vi "数据编码.vi"(0 "table输入":string(combo), 1 "仪器参数上传时间":enum16{"精确到小时", "原始时间"}(ring), 5 "错误常量 2":errorcluster caption="错误输入", 7 "仪器参数":string[](array[string]), 9 "QN":string, 11 "参数":string, 13 "MN":string, 14 "PW":string) -> (4 "错误常量":errorcluster caption="错误输出", 15 "通讯包字符串":string)   [LabVIEW 2016, in "数据传输系统-06.lvlib"]
panel:
  out "核查数据发送次数":i32
  out "小时数据发送次数":i32
  out "长度":i32
  in  "数据块":T1
  out "通讯包":T2={"包头（2）"="##", "数据段长度（4）"="", "数据段"="", "CRC校验"="", "包尾"=""}
  # "范例代码：\n\n##0101QN=20160801085857223;ST=32;CN=1062;PW=100000;MN=010000A8900016F000169DC0;Flag=5\n;CP=&&RtdInterval=30&&1C80\\r\\n"
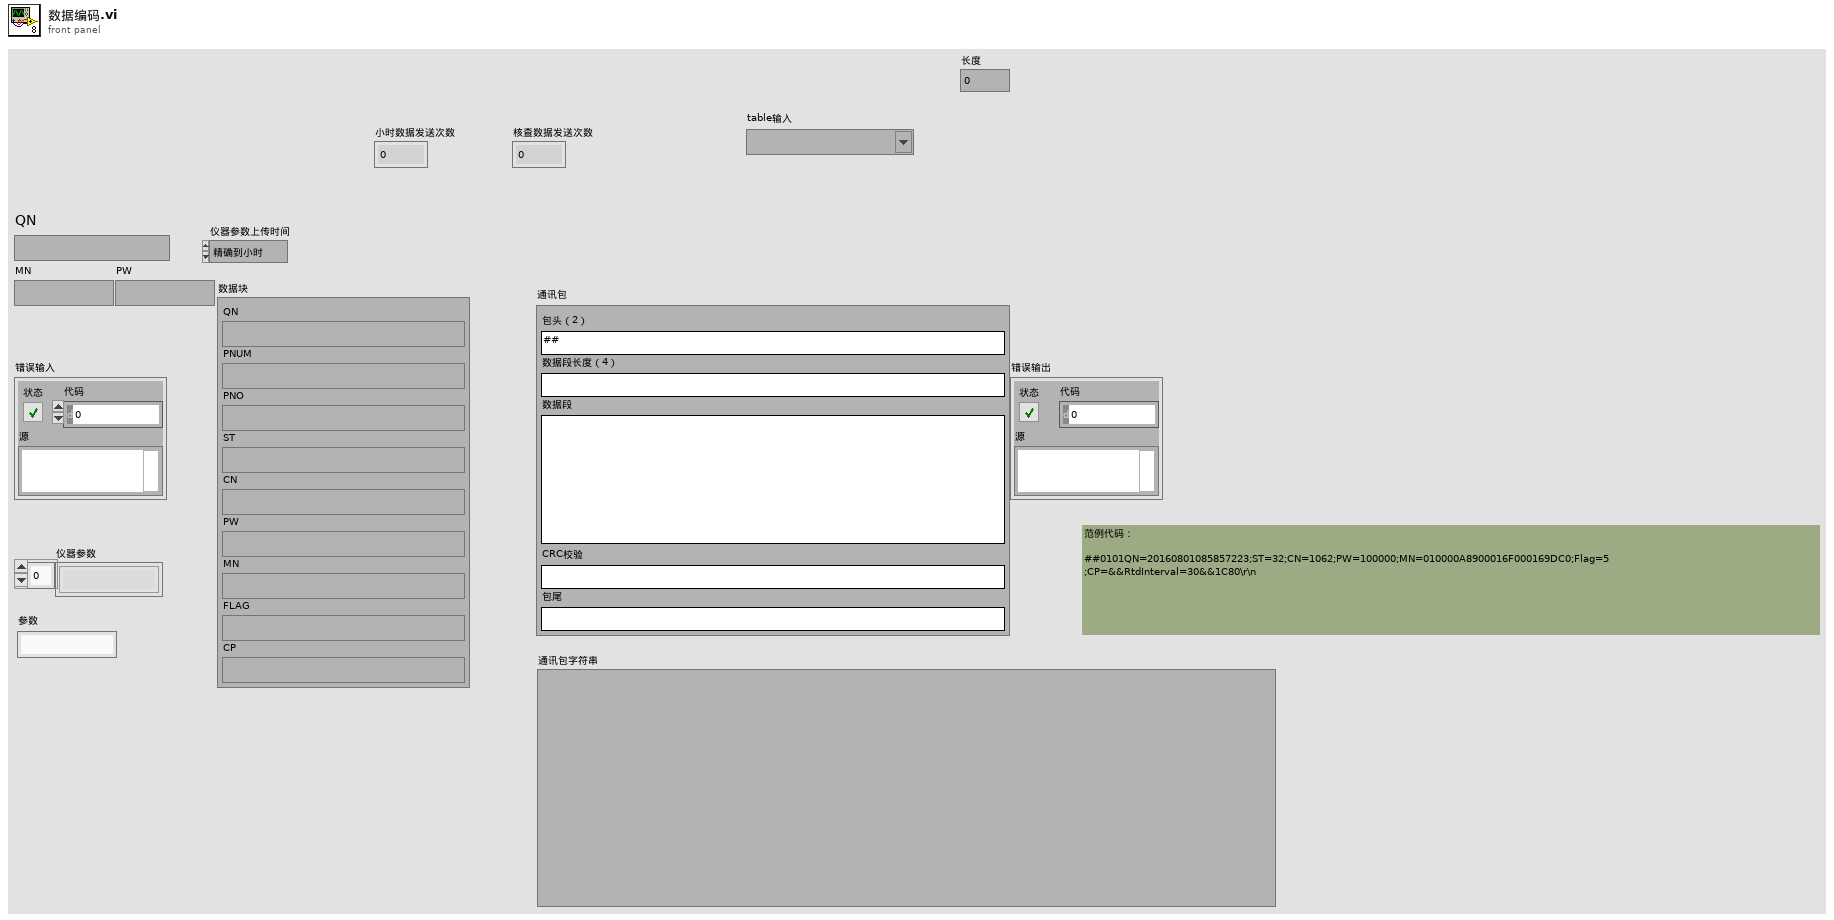
[diagram p1: front panel]
types:
  T1 = cluster{"QN":string, "ST":string, "CN":string, "PW":string, "MN":string, "FLAG":string, "PNUM":string, "PNO":string, "CP":string}
  T2 = cluster{"包头（2）":string, "数据段长度（4）":string, "数据段":string, "CRC校验":string, "包尾":string}
  T3 = cluster{"PH":string[][], "CODCr":string[][], "氨氮":string[][], "CODMn":string[][], "总氮":string[][], "总磷":string[][], "电导率":string[][], "水温":string[][], "DO":string[][], "浊度":string[][], "叶绿素":string[][], "藻密度":string[][], "铜":string[][], "盐度":string[][], "水位":string[][], "流速":string[][], "瞬时流量":string[][], "累积流量":string[][], "亚硝酸盐":string[][], "硫化物":string[][], "ORP":string[][], "铅":string[][], "镉":string[][], "锌":string[][], "镍":string[][], "锰":string[][], "汞":string[][], "气温":string[][], "气压":string[][], "风速":string[][], "风向":string[][], "盐度 2":string[][], "磷酸盐":string[][], "硝氮":string[][], "氟化物":string[][], "挥发酚":string[][], "氯化物":string[][]}
  T4 = enum16{"小时数据", "实时数据", "平行样测试", "集成干预测试", "加标回收测试", "核查数据", "空白零点跨度数据", "提取小时数据", "提取实时数据"}
  T5 = enum16{"小时数据", "实时数据", "平行样测试", "集成干预测试", "加标回收测试", "核查数据", "空白零点跨度数据", "提取小时数据", "提取实时数据", "操作日志"}
  T6 = enum16{"小时数据", "实时数据", "平行样测试", "集成干预测试", "加标回收测试", "核查数据", "空白零点跨度数据", "提取小时数据", "提取实时数据", "操作日志", "仪器参数", "3090仪器参数", "提取仪器参数", "报警信息"}
  T7 = cluster{"CODMn固件信息":string, "氨氮固件信息":string, "总磷固件信息":string, "总氮固件信息":string, "CODCr固件信息":string}
  T8 = typedef "数据传输系统-06.lvlib/应用环境.ctl" = enum16{"STD", "GB212", "婉仪平台"}
  T9 = cluster{"CODMn":dbl, "CODCr":dbl, "DO":dbl, "铜":dbl, "PH":dbl, "氨氮":dbl, "比电导率":dbl, "水温":dbl, "COD":dbl, "浊度":dbl, "总氮":dbl, "总磷":dbl, "叶绿素a":dbl, "藻密度":dbl, "水位":dbl, "流速":dbl, "瞬时流量":dbl, "累积流量":dbl, "亚硝酸盐":dbl, "硫化物":dbl, "ORP":dbl, "铅":dbl, "镉":dbl, "锌":dbl, "镍":dbl, "锰":dbl, "汞":dbl, "气温":dbl, "气压":dbl, "风速":dbl, "风向":dbl, "盐度":dbl, "磷酸盐":dbl, "硝氮":dbl, "氟化物":dbl, "挥发酚":dbl, "氯化物":dbl}
  T10 = cluster{"CODMn":string, "CODCr":string, "DO":string, "铜":string, "PH":string, "氨氮":string, "比电导率":string, "水温":string, "COD":string, "浊度":string, "总氮":string, "总磷":string, "叶绿素a":string, "藻密度":string, "水位":string, "流速":string, "瞬时流量":string, "累积流量":string, "亚硝酸盐":string, "硫化物":string, "ORP":string, "铅":string, "镉":string, "锌":string, "镍":string, "锰":string, "汞":string, "气温":string, "气压":string, "风速":string, "风向":string, "盐度":string, "磷酸盐":string, "硝氮":string, "氟化物":string, "挥发酚":string, "氯化物":string}
  T11 = typedef "LVDateTimeRec.ctl" = cluster{"秒数的小数部分":dbl, "秒":i32, "分":i32, "时":i32, "日":i32, "月":i32, "年":i32, "天数（周）":i32, "天数（年）":i32, "DST":i32}
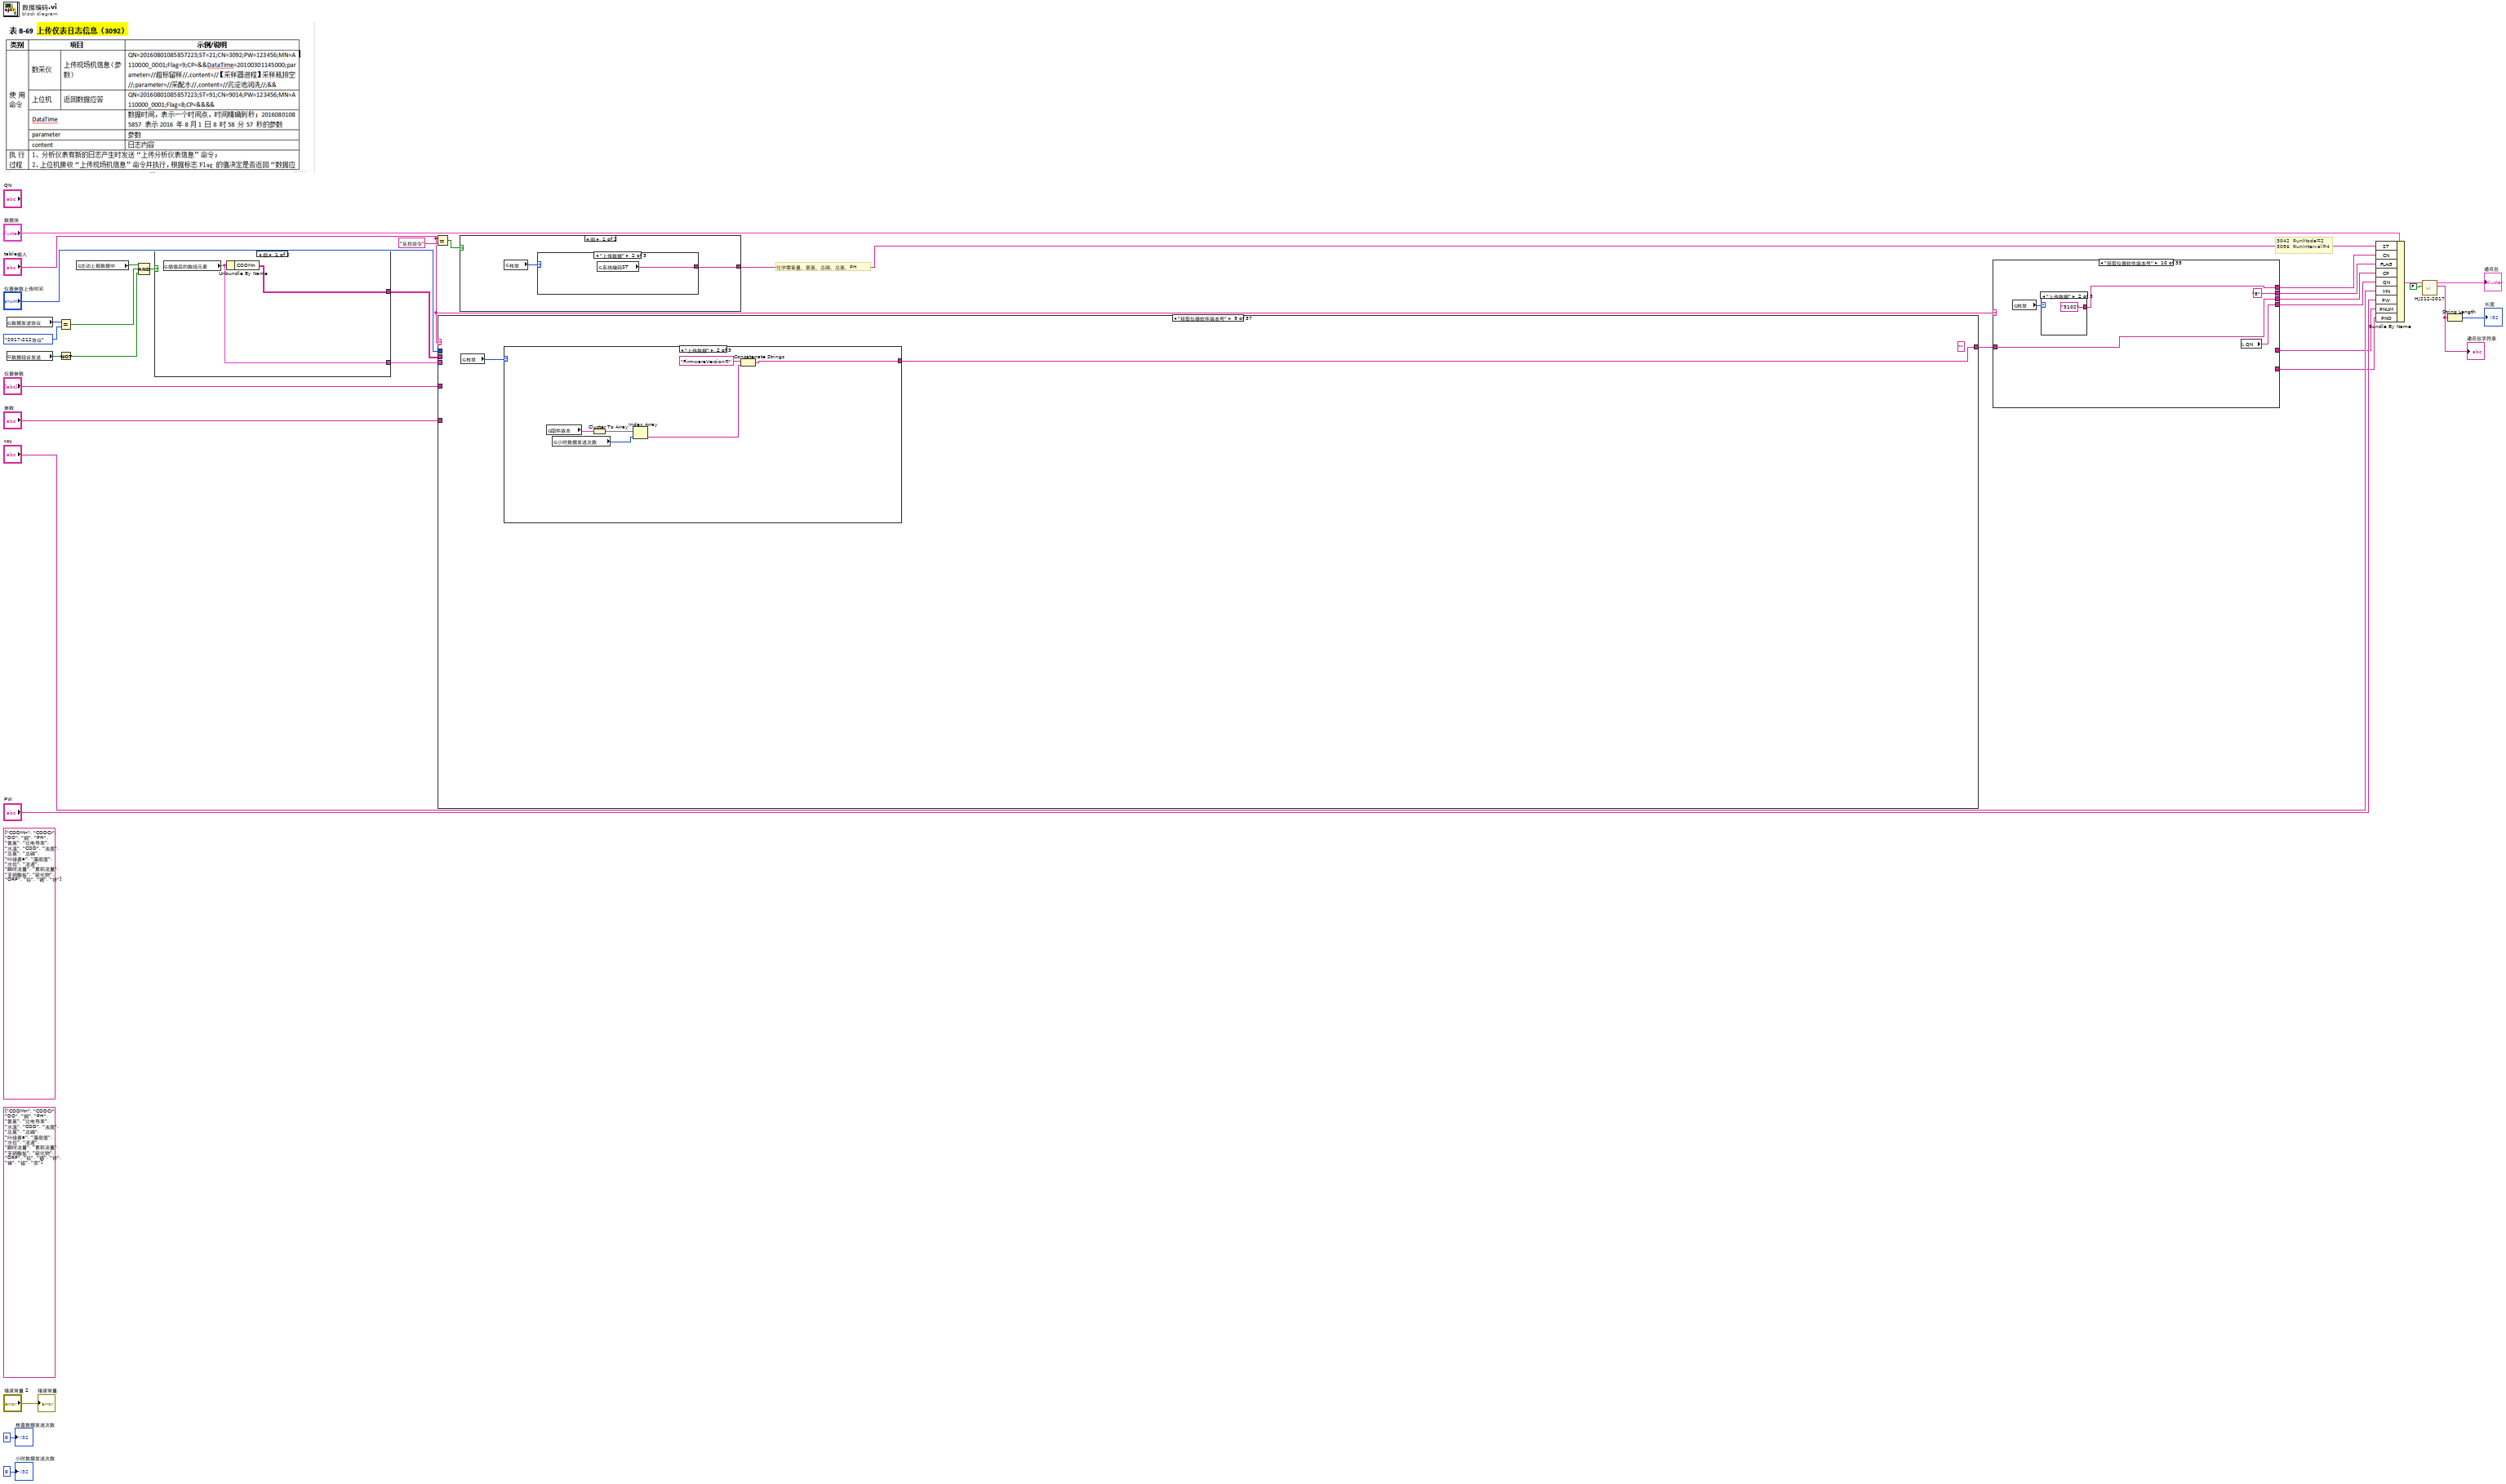
[diagram p0: block diagram]
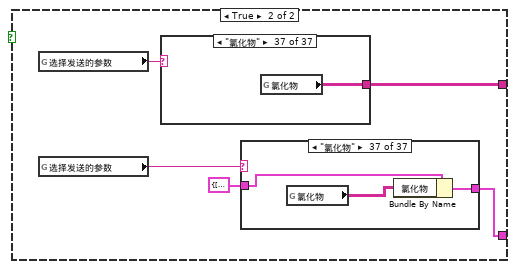
[diagram p2: hidden frame]
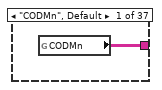
[diagram p3: hidden frame]
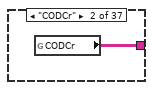
[diagram p4: hidden frame]
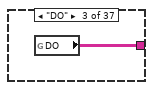
[diagram p5: hidden frame]
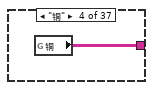
[diagram p6: hidden frame]
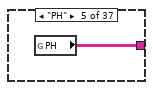
[diagram p7: hidden frame]
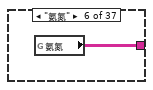
[diagram p8: hidden frame]
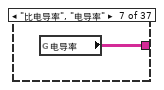
[diagram p9: hidden frame]
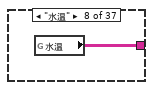
[diagram p10: hidden frame]
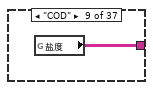
[diagram p11: hidden frame]
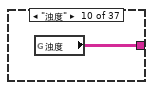
[diagram p12: hidden frame]
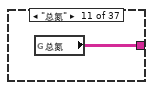
[diagram p13: hidden frame]
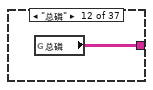
[diagram p14: hidden frame]
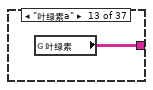
[diagram p15: hidden frame]
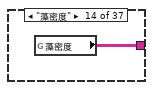
[diagram p16: hidden frame]
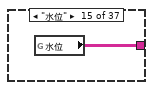
[diagram p17: hidden frame]
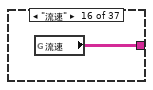
[diagram p18: hidden frame]
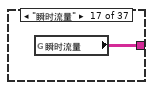
[diagram p19: hidden frame]
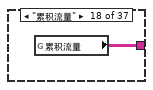
[diagram p20: hidden frame]
diagram:
  (unwired) string[] ["CODMn", "CODCr", "DO", "铜", "PH", "氨氮", "比电导率", "水温", "COD", "浊度", "总氮", "总磷", "叶绿素a", "藻密度", "水位", "流速", "瞬时流量", "累积流量", "亚硝酸盐", "硫化物", "ORP", "铅", "镉", "锌"] ("数组")
  (unwired) string[] ["CODMn", "CODCr", "DO", "铜", "PH", "氨氮", "比电导率", "水温", "COD", "浊度", "总氮", "总磷", "叶绿素a", "藻密度", "水位", "流速", "瞬时流量", "累积流量", "亚硝酸盐", "硫化物", "ORP", "铅", "镉", "锌", "镍", "锰", "汞"] ("数组")
  # "化学需氧量、氨氮、总磷、总氮、PH"
  # "3042  RunMode=2\n3056  RunInterval=4"
  n1 = global read "断电保存全局.vi" "数据发送协议"() -> (w11:enum16{"2005-212协议", "2017-212协议"})
  n2 = global read "断电保存全局.vi" "数据组合发送"() -> (w13:bool)
  n3 = Equal?(x=w11, y=enum16{"2005-212协议", "2017-212协议"}."2017-212协议" ("数据发送版本")) -> (x = y?=w14:bool)
  n4 = Not(x=w13) -> (.not. x?=w12:bool)
  n5 = global read "全局 数据发送重叠.vi" "主动上报数据中"() -> (w18:bool)
  n6 = Compound Arithmetic op=AND ("复合运算")(w18, w14, w12) -> (w15:bool)
  n7 = case shown="假" w15 {
    tunnel: [w36 w40] -> w9
    tunnel: [w35 w38] -> w7
    frame False {
      n8 = global read "插值后的新数组.vi" "插值后的数组元素"() -> (w36:T3)
      n9 = Unbundle By Name(w36) -> ("CODMn"=w35:string[][])
    }
    frame True {
      n10 = global read "全局 水样时间.vi" "选择发送的参数"() -> (w39:string)
      n11 = global read "全局 水样时间.vi" "选择发送的参数"() -> (w41:string)
      n12 = case shown="\"氯化物\"" w39 {
        tunnel: [w42 w43 w44 w45 w46 w47 w48 w49 w50 w51 w52 w53 w54 w55 w56 w57 w58 w59 w60 w61 w62 w63 w64 w65 w66 w67 w68 w69 w70 w71 w72 w73 w74 w75 w76 w77 w78] -> w38
        frame "CODMn", Default {
          n13 = global read "全局 所有参数.vi" "CODMn"() -> (w42:string[][])
        }
        frame "CODCr" {
          n14 = global read "全局 所有参数.vi" "CODCr"() -> (w43:string[][])
        }
        frame "DO" {
          n15 = global read "全局 所有参数.vi" "DO"() -> (w44:string[][])
        }
        frame "铜" {
          n16 = global read "全局 所有参数.vi" "铜"() -> (w45:string[][])
        }
        frame "PH" {
          n17 = global read "全局 所有参数.vi" "PH"() -> (w46:string[][])
        }
        frame "氨氮" {
          n18 = global read "全局 所有参数.vi" "氨氮"() -> (w47:string[][])
        }
        frame "比电导率", "电导率" {
          n19 = global read "全局 所有参数.vi" "电导率"() -> (w48:string[][])
        }
        frame "水温" {
          n20 = global read "全局 所有参数.vi" "水温"() -> (w49:string[][])
        }
        frame "COD" {
          n21 = global read "全局 所有参数.vi" "盐度"() -> (w50:string[][])
        }
        frame "浊度" {
          n22 = global read "全局 所有参数.vi" "浊度"() -> (w51:string[][])
        }
        frame "总氮" {
          n23 = global read "全局 所有参数.vi" "总氮"() -> (w52:string[][])
        }
        frame "总磷" {
          n24 = global read "全局 所有参数.vi" "总磷"() -> (w53:string[][])
        }
        frame "叶绿素a" {
          n25 = global read "全局 所有参数.vi" "叶绿素"() -> (w54:string[][])
        }
        frame "藻密度" {
          n26 = global read "全局 所有参数.vi" "藻密度"() -> (w55:string[][])
        }
        frame "水位" {
          n27 = global read "全局 所有参数.vi" "水位"() -> (w56:string[][])
        }
        frame "流速" {
          n28 = global read "全局 所有参数.vi" "流速"() -> (w57:string[][])
        }
        frame "瞬时流量" {
          n29 = global read "全局 所有参数.vi" "瞬时流量"() -> (w58:string[][])
        }
        frame "累积流量" {
          n30 = global read "全局 所有参数.vi" "累积流量"() -> (w59:string[][])
        }
        frame "亚硝氮" {
          n31 = global read "全局 所有参数.vi" "亚硝酸盐"() -> (w60:string[][])
        }
        frame "硫化物" {
          n32 = global read "全局 所有参数.vi" "硫化物"() -> (w61:string[][])
        }
        frame "ORP" {
          n33 = global read "全局 所有参数.vi" "ORP"() -> (w62:string[][])
        }
        frame "铅" {
          n34 = global read "全局 所有参数.vi" "铅"() -> (w63:string[][])
        }
        frame "镉" {
          n35 = global read "全局 所有参数.vi" "镉"() -> (w64:string[][])
        }
        frame "锌" {
          n36 = global read "全局 所有参数.vi" "锌"() -> (w65:string[][])
        }
        frame "镍" {
          n37 = global read "全局 所有参数.vi" "镍"() -> (w66:string[][])
        }
        frame "锰" {
          n38 = global read "全局 所有参数.vi" "锰"() -> (w67:string[][])
        }
        frame "汞" {
          n39 = global read "全局 所有参数.vi" "汞"() -> (w68:string[][])
        }
        frame "气温" {
          n40 = global read "全局 所有参数.vi" "气温"() -> (w69:string[][])
        }
        frame "气压" {
          n41 = global read "全局 所有参数.vi" "气压"() -> (w70:string[][])
        }
        frame "风速" {
          n42 = global read "全局 所有参数.vi" "风速"() -> (w71:string[][])
        }
        frame "风向" {
          n43 = global read "全局 所有参数.vi" "风向"() -> (w72:string[][])
        }
        frame "盐度" {
          n44 = global read "全局 所有参数.vi" "盐度 2"() -> (w73:string[][])
        }
        frame "磷酸盐" {
          n45 = global read "全局 所有参数.vi" "磷酸盐"() -> (w74:string[][])
        }
        frame "硝氮" {
          n46 = global read "全局 所有参数.vi" "硝氮"() -> (w75:string[][])
        }
        frame "氟化物" {
          n47 = global read "全局 所有参数.vi" "氟化物"() -> (w76:string[][])
        }
        frame "挥发酚" {
          n48 = global read "全局 所有参数.vi" "挥发酚"() -> (w77:string[][])
        }
        frame "氯化物" {
          n49 = global read "全局 所有参数.vi" "氯化物"() -> (w78:string[][])
        }
      }
      n50 = case shown="\"氯化物\"" w41 {
        tunnel: T3 {"PH"=[], "CODCr"=[], "氨氮"=[], "CODMn"=[], "总氮"=[], "总磷"=[], "电导率"=[], "水温"=[], "DO"=[], "浊度"=[], "叶绿素"=[], "藻密度"=[], "铜"=[], "盐度"=[], "水位"=[], "流速"=[], "瞬时流量"=[], "累积流量"=[], "亚硝酸盐"=[], "硫化物"=[], "ORP"=[], "铅"=[], "镉"=[], "锌"=[], "镍"=[], "锰"=[], "汞"=[], "气温"=[], "气压"=[], "风速"=[], "风向"=[], "盐度 2"=[], "磷酸盐"=[], "硝氮"=[], "氟化物"=[], "挥发酚"=[], "氯化物"=[]} ("插值后的数组元素") -> [w80 w84 w87 w90 w93 w96 w99 w102 w105 w108 w111 w114 w117 w119 w123 w126 w128 w131 w134 w137 w140 w143 w146 w149 w152 w155 w158 w161 w164 w167 w170 w173 w176 w179 w182 w185 w188]
        tunnel: [w79 w82 w85 w88 w91 w94 w98 w101 w103 w106 w109 w112 w115 w118 w121 w124 w127 w130 w133 w136 w139 w142 w145 w148 w151 w154 w157 w160 w163 w166 w169 w172 w175 w178 w181 w184 w187] -> w40
        frame "CODMn", Default {
          n51 = global read "全局 所有参数.vi" "CODMn"() -> (w81:string[][])
          n52 = Bundle By Name(cluster=w80, "CODMn"=w81) -> (w79:T3)
        }
        frame "CODCr" {
          n53 = global read "全局 所有参数.vi" "CODCr"() -> (w83:string[][])
          n54 = Bundle By Name(cluster=w84, "CODCr"=w83) -> (w82:T3)
        }
        frame "DO" {
          n55 = global read "全局 所有参数.vi" "DO"() -> (w86:string[][])
          n56 = Bundle By Name(cluster=w87, "DO"=w86) -> (w85:T3)
        }
        frame "铜" {
          n57 = global read "全局 所有参数.vi" "铜"() -> (w89:string[][])
          n58 = Bundle By Name(cluster=w90, "铜"=w89) -> (w88:T3)
        }
        frame "PH" {
          n59 = global read "全局 所有参数.vi" "PH"() -> (w92:string[][])
          n60 = Bundle By Name(cluster=w93, "PH"=w92) -> (w91:T3)
        }
        frame "氨氮" {
          n61 = global read "全局 所有参数.vi" "氨氮"() -> (w95:string[][])
          n62 = Bundle By Name(cluster=w96, "氨氮"=w95) -> (w94:T3)
        }
        frame "比电导率", "电导率" {
          n63 = global read "全局 所有参数.vi" "电导率"() -> (w97:string[][])
          n64 = Bundle By Name(cluster=w99, "电导率"=w97) -> (w98:T3)
        }
        frame "水温" {
          n65 = global read "全局 所有参数.vi" "水温"() -> (w100:string[][])
          n66 = Bundle By Name(cluster=w102, "水温"=w100) -> (w101:T3)
        }
        frame "COD" {
          n67 = global read "全局 所有参数.vi" "盐度"() -> (w104:string[][])
          n68 = Bundle By Name(cluster=w105, "盐度"=w104) -> (w103:T3)
        }
        frame "浊度" {
          n69 = global read "全局 所有参数.vi" "浊度"() -> (w107:string[][])
          n70 = Bundle By Name(cluster=w108, "浊度"=w107) -> (w106:T3)
        }
        frame "总氮" {
          n71 = global read "全局 所有参数.vi" "总氮"() -> (w110:string[][])
          n72 = Bundle By Name(cluster=w111, "总氮"=w110) -> (w109:T3)
        }
        frame "总磷" {
          n73 = global read "全局 所有参数.vi" "总磷"() -> (w113:string[][])
          n74 = Bundle By Name(cluster=w114, "总磷"=w113) -> (w112:T3)
        }
        frame "叶绿素a" {
          n75 = global read "全局 所有参数.vi" "叶绿素"() -> (w116:string[][])
          n76 = Bundle By Name(cluster=w117, "叶绿素"=w116) -> (w115:T3)
        }
        frame "藻密度" {
          n77 = global read "全局 所有参数.vi" "藻密度"() -> (w120:string[][])
          n78 = Bundle By Name(cluster=w119, "藻密度"=w120) -> (w118:T3)
        }
        frame "水位" {
          n79 = global read "全局 所有参数.vi" "水位"() -> (w122:string[][])
          n80 = Bundle By Name(cluster=w123, "水位"=w122) -> (w121:T3)
        }
        frame "流速" {
          n81 = global read "全局 所有参数.vi" "流速"() -> (w125:string[][])
          n82 = Bundle By Name(cluster=w126, "流速"=w125) -> (w124:T3)
        }
        frame "瞬时流量" {
          n83 = global read "全局 所有参数.vi" "瞬时流量"() -> (w129:string[][])
          n84 = Bundle By Name(cluster=w128, "瞬时流量"=w129) -> (w127:T3)
        }
        frame "累积流量" {
          n85 = global read "全局 所有参数.vi" "累积流量"() -> (w132:string[][])
          n86 = Bundle By Name(cluster=w131, "累积流量"=w132) -> (w130:T3)
        }
        frame "亚硝氮" {
          n87 = global read "全局 所有参数.vi" "亚硝酸盐"() -> (w135:string[][])
          n88 = Bundle By Name(cluster=w134, "亚硝酸盐"=w135) -> (w133:T3)
        }
        frame "硫化物" {
          n89 = global read "全局 所有参数.vi" "硫化物"() -> (w138:string[][])
          n90 = Bundle By Name(cluster=w137, "硫化物"=w138) -> (w136:T3)
        }
        frame "ORP" {
          n91 = global read "全局 所有参数.vi" "ORP"() -> (w141:string[][])
          n92 = Bundle By Name(cluster=w140, "ORP"=w141) -> (w139:T3)
        }
        frame "铅" {
          n93 = global read "全局 所有参数.vi" "铅"() -> (w144:string[][])
          n94 = Bundle By Name(cluster=w143, "铅"=w144) -> (w142:T3)
        }
        frame "镉" {
          n95 = global read "全局 所有参数.vi" "镉"() -> (w147:string[][])
          n96 = Bundle By Name(cluster=w146, "镉"=w147) -> (w145:T3)
        }
        frame "锌" {
          n97 = global read "全局 所有参数.vi" "锌"() -> (w150:string[][])
          n98 = Bundle By Name(cluster=w149, "锌"=w150) -> (w148:T3)
        }
        frame "镍" {
          n99 = global read "全局 所有参数.vi" "镍"() -> (w153:string[][])
          n100 = Bundle By Name(cluster=w152, "镍"=w153) -> (w151:T3)
        }
        frame "锰" {
          n101 = global read "全局 所有参数.vi" "锰"() -> (w156:string[][])
          n102 = Bundle By Name(cluster=w155, "锰"=w156) -> (w154:T3)
        }
        frame "汞" {
          n103 = global read "全局 所有参数.vi" "汞"() -> (w159:string[][])
          n104 = Bundle By Name(cluster=w158, "汞"=w159) -> (w157:T3)
        }
        frame "气温" {
          n105 = global read "全局 所有参数.vi" "气温"() -> (w162:string[][])
          n106 = Bundle By Name(cluster=w161, "气温"=w162) -> (w160:T3)
        }
        frame "气压" {
          n107 = global read "全局 所有参数.vi" "气压"() -> (w165:string[][])
          n108 = Bundle By Name(cluster=w164, "气压"=w165) -> (w163:T3)
        }
        frame "风速" {
          n109 = global read "全局 所有参数.vi" "风速"() -> (w168:string[][])
          n110 = Bundle By Name(cluster=w167, "风速"=w168) -> (w166:T3)
        }
        frame "风向" {
          n111 = global read "全局 所有参数.vi" "风向"() -> (w171:string[][])
          n112 = Bundle By Name(cluster=w170, "风向"=w171) -> (w169:T3)
        }
        frame "盐度" {
          n113 = global read "全局 所有参数.vi" "盐度 2"() -> (w174:string[][])
          n114 = Bundle By Name(cluster=w173, "盐度 2"=w174) -> (w172:T3)
        }
        frame "磷酸盐" {
          n115 = global read "全局 所有参数.vi" "磷酸盐"() -> (w177:string[][])
          n116 = Bundle By Name(cluster=w176, "磷酸盐"=w177) -> (w175:T3)
        }
        frame "硝氮" {
          n117 = global read "全局 所有参数.vi" "硝氮"() -> (w180:string[][])
          n118 = Bundle By Name(cluster=w179, "硝氮"=w180) -> (w178:T3)
        }
        frame "氟化物" {
          n119 = global read "全局 所有参数.vi" "氟化物"() -> (w183:string[][])
          n120 = Bundle By Name(cluster=w182, "氟化物"=w183) -> (w181:T3)
        }
        frame "挥发酚" {
          n121 = global read "全局 所有参数.vi" "挥发酚"() -> (w186:string[][])
          n122 = Bundle By Name(cluster=w185, "挥发酚"=w186) -> (w184:T3)
        }
        frame "氯化物" {
          n123 = global read "全局 所有参数.vi" "氯化物"() -> (w189:string[][])
          n124 = Bundle By Name(cluster=w188, "氯化物"=w189) -> (w187:T3)
        }
      }
    }
  }
  n125 = Equal?(x="table输入", y="反控命令") -> (x = y?=w24:bool)
  n126 = case shown="\"获取仪器软件版本号\"" "table输入" {
    tunnel: [w191 w198 w212 w254 w292 _ w306 w315 w322 w332 w343 w493 w524 w575 w623 w675 w704 w736 w767 w793 w822 w851 w888 w921 w954 w993 w1154 w1196 w1357 w1385 w1408 w1441 w1464 w1475 w1483 w1493 w1503] -> w19
    tunnel: w7 -> [_ _ _ _ _ _ _ _ _ _ w340 w492 _ _ _ w674 w705 w731 w762 w794 w821 w850 w887 _ _ _ _ _ w1356 _ w1407 _ _ _ _ _ _]
    tunnel: w9 -> [_ _ _ _ _ _ _ _ _ _ w341 w494 _ _ _ w670 w700 w732 w763 w792 w820 w849 w883 _ _ _ _ _ w1352 w1383 w1403 _ _ _ _ _ _]
    tunnel: "仪器参数" -> [_ _ _ _ _ _ _ _ _ _ _ _ _ _ _ _ _ _ _ _ _ _ _ _ _ w989 w1152 w1192 _ _ _ _ _ _ _ _ _]
    tunnel: "参数" -> [_ _ _ _ _ _ _ _ _ _ _ _ _ _ _ _ _ _ _ _ _ _ _ _ _ w991 _ w1194 _ _ _ _ _ _ _ _ _]
    tunnel: "仪器参数上传时间" -> [_ _ _ _ _ _ _ _ _ _ _ _ _ _ _ _ _ _ _ _ _ _ _ _ _ w988 w1151 w1191 _ _ _ _ _ _ _ _ _]
    frame "反控命令" {
      n127 = global read "全局 反控命令枚举.vi" "反控命令枚举"() -> (w190:enum16{"返回请求应答", "返回执行结果"})
      n128 = case shown="\"返回执行结果\"" w190 {
        tunnel: ["QnRtn=1" w194] -> w191
        frame "返回请求应答", Default {
        }
        frame "返回执行结果" {
          n129 = global read "全局 反控命令枚举.vi" "执行结果定义"() -> (w195:u16)
          n130 = Number To Decimal String(number=w195) -> (decimal integer string=w193:string)  [unwired: 1 in]
          n131 = Concatenate Strings("ExeRtn=", w193) -> (w194:string)
        }
      }
    }
    frame "超标留样返回" {
      n132 = global read "全局1.vi" "枚举"() -> (w197:enum16{"返回请求应答", "上传数据", "返回执行结果"})
      n133 = case shown="\"返回执行结果\"" w197 {
        tunnel: ["QnRtn=1" w200 "ExeRtn=1"] -> w198
        frame "返回请求应答", Default {
        }
        frame "上传数据" {
          n134 = global read "全局1.vi" "register values"() -> (w209:u16[])
          n135 = Get Date/Time In Seconds() -> (seconds since 1Jan1904=w207:timestamp)
          n136 = Index Array(array=w209, index=7 ("索引")) -> (element=w202:u16)
          n137 = Format Date/Time String(time format string (%c)="%Y%m%d%H%M%S" ("时间格式字符串(%c)"), seconds (now)=w207) -> (date/time string=w205:string)  [unwired: 1 in]
          n138 = Number To Decimal String(number=w202) -> (decimal integer string=w203:string)  [unwired: 1 in]
          n139 = Format Into String(format string="VaseNo=%s" ("格式字符串"), w203) -> (resulting string=w201:string)  [unwired: 2 in, 1 out]
          n140 = Format Into String(format string="DataTime=%s;%s" ("格式字符串"), w205, w201) -> (resulting string=w200:string)  [unwired: 2 in, 1 out]
        }
        frame "返回执行结果" {
        }
      }
    }
    frame "提取经纬度环境信息" {
      # "BDS纬度"
      # "BDS纬度"
      # "GPS纬度"
      # "GPS经度"
      # "湿度"
      # "温度"
      # "电压"
      # "时间"
      n141 = global read "全局1.vi" "枚举"() -> (w213:enum16{"返回请求应答", "上传数据", "返回执行结果"})
      n142 = case shown="\"上传数据\"" w213 {
        tunnel: ["QnRtn=1" w226 "ExeRtn=1"] -> w212
        frame "返回请求应答", Default {
        }
        frame "上传数据" {
          n143 = global read "全局 环境参数.vi" "环境参数"() -> (w216:string[][])
          n144 = global read "全局 环境参数.vi" "columns输出"() -> (w223:string[])
          n145 = Index Array(array=w216, index (row)=0 ("索引 (行)")) -> (element=w219:string[])  [unwired: 1 in]
          n146 = Get Date/Time In Seconds() -> (seconds since 1Jan1904=w228:timestamp)
          n147 = Array Subset(array=w223, index=1 ("索引")) -> (w224:string[])  [unwired: 1 in]
          n148 = for {
            tunnel: w224 -> [w232] mode=indexing
            tunnel: [w231] -> w225 mode=indexing
            n149 = case shown="\"BDS经度\"" w232 {
              tunnel: ["" "Volt=%s;" "Temp=%s;" ("格式字符串") "Hum=%s;" ("格式字符串") "Lng=%s;" "Lat=%s;" "Lng2=%s;" "Lat2=%s;"] -> w231
              frame "假", Default {
              }
              frame "电压" {
              }
              frame "室温" {
              }
              frame "湿度" {
              }
              frame "GPS经度" {
              }
              frame "GPS纬度" {
              }
              frame "BDS经度" {
              }
              frame "BDS纬度" {
              }
            }
          }
          n150 = Format Date/Time String(time format string (%c)="%Y%m%d%H%M%S" ("时间格式字符串(%c)"), seconds (now)=w228) -> (date/time string=w227:string)  [unwired: 1 in]
          n151 = Array Subset(array=w219, index=1 ("索引")) -> (w221:string[])  [unwired: 1 in]
          n152 = for {
            shift-right: [w246] -> w215
            shift-left: "" -> [w245]
            tunnel: w225 -> [w244] mode=indexing
            tunnel: w221 -> [w242] mode=indexing
            n153 = Empty String/Path?(string/path=w242) -> (empty?=w248:bool)
            n154 = Fract/Exp String To Number(string=w242) -> (number=w243:dbl)  [unwired: 3 in, 1 out]
            n155 = Number To Fractional String(number=w243) -> (F-format string=w241:string)  [unwired: 3 in]
            n156 = case shown="假" w248 {
              tunnel: [w251 w252] -> w247
              tunnel: w244 -> [w250 _]
              tunnel: w241 -> [w249 _]
              tunnel: w241 -> [_ w252]
              frame False {
                n157 = Format Into String(format string=w250, w249) -> (resulting string=w251:string)  [unwired: 2 in, 1 out]
              }
              frame True {
              }
            }
            n158 = Concatenate Strings(w245, w247) -> (w246:string)
          }
          n159 = Format Into String(format string="DataTime=%s;%s" ("格式字符串"), w227, w215) -> (resulting string=w226:string)  [unwired: 2 in, 1 out]
        }
        frame "返回执行结果" {
        }
      }
    }
    frame "提取现场系统信息" {
      n160 = global read "全局1.vi" "枚举"() -> (w255:enum16{"返回请求应答", "上传数据", "返回执行结果"})
      n161 = case shown="\"上传数据\"" w255 {
        tunnel: ["QnRtn=1" w289 "ExeRtn=1"] -> w254
        frame "返回请求应答", Default {
        }
        frame "上传数据" {
          n162 = global read "全局1.vi" "register values"() -> (w288:u16[])
          n163 = global read "全局1.vi" "系统信息"() -> (w270:u16[])
          n164 = Get Date/Time In Seconds() -> (seconds since 1Jan1904=w275:timestamp)
          n165 = Format Date/Time String(time format string (%c)="%Y%m%d%H%M%S%u" ("时间格式字符串(%c)"), seconds (now)=w275) -> (date/time string=w278:string)  [unwired: 1 in]
          n166 = Number To Decimal String(number=w270) -> (decimal integer string=w269:string[])  [unwired: 1 in]
          n167 = Index Array(array=w288, index #1=0 ("索引"), index #2=6 ("索引")) -> (element #1=w284:u16, element #2=w272:u16)
          n168 = Number To Decimal String(number=w284) -> (decimal integer string=w286:string)  [unwired: 1 in]
          n169 = Number To Decimal String(number=w272) -> (decimal integer string=w281:string)  [unwired: 1 in]
          n170 = Index Array(array=w269) -> (element #1=w267:string, element #2=w264:string, element #3=w261:string, element #4=w258:string)  [unwired: 4 in]
          n171 = Search and Replace String(input string=w278, search string="." ("搜索字符串")) -> (result string=w274:string)  [unwired: 6 in, 3 out]
          n172 = Format Into String(format string="SystemTask=%s;" ("格式字符串"), w267) -> (resulting string=w266:string)  [unwired: 2 in, 1 out]
          n173 = Format Into String(format string="PumpState=%s;" ("格式字符串"), w264) -> (resulting string=w263:string)  [unwired: 2 in, 1 out]
          n174 = Format Into String(format string="AlgClean=%s;" ("格式字符串"), w261) -> (resulting string=w260:string)  [unwired: 2 in, 1 out]
          n175 = Format Into String(format string="SystemAlarm=0%s;" ("格式字符串"), w258) -> (resulting string=w257:string)  [unwired: 2 in, 1 out]
          n176 = Format Into String(format string="RunMode=%s;" ("格式字符串"), w286) -> (resulting string=w271:string)  [unwired: 2 in, 1 out]
          n177 = Format Into String(format string="RunInterval=%s;" ("格式字符串"), w281) -> (resulting string=w282:string)  [unwired: 2 in, 1 out]
          n178 = Format Into String(format string="SystemTime=%s;" ("格式字符串"), w274) -> (resulting string=w279:string)  [unwired: 2 in, 1 out]
          n179 = Concatenate Strings(w271, w263, w266, w260, w257, w282, w279) -> (w289:string)
        }
        frame "返回执行结果" {
        }
      }
    }
    frame "提取监测仪表时间" {
      n180 = global read "全局1.vi" "枚举"() -> (w291:enum16{"返回请求应答", "上传数据", "返回执行结果"})
      n181 = case shown="\"上传数据\"" w291 {
        tunnel: ["QnRtn=1" w304 "ExeRtn=1"] -> w292
        frame "返回请求应答", Default {
        }
        frame "上传数据" {
          n182 = global read "全局 提取仪器参数.vi" "仪器编码"() -> (w294:string)
          n183 = Format Into String(format string="PolId=%s;" ("格式字符串"), w294) -> (resulting string=w302:string)  [unwired: 2 in, 1 out]
          n184 = Get Date/Time In Seconds() -> (seconds since 1Jan1904=w297:timestamp)
          n185 = Format Date/Time String(time format string (%c)="%Y%m%d%H%M%S%u" ("时间格式字符串(%c)"), seconds (now)=w297) -> (date/time string=w300:string)  [unwired: 1 in]
          n186 = Search and Replace String(input string=w300, search string="." ("搜索字符串")) -> (result string=w296:string)  [unwired: 6 in, 3 out]
          n187 = Format Into String(format string="SystemTime=%s;" ("格式字符串"), w296) -> (resulting string=w295:string)  [unwired: 2 in, 1 out]
          n188 = Concatenate Strings(w302, w295) -> (w304:string)
        }
        frame "返回执行结果" {
        }
      }
    }
    frame "心跳包", Default {
    }
    frame "提取数采仪时间" {
      (unwired) ""
      n189 = global read "全局1.vi" "枚举"() -> (w307:enum16{"返回请求应答", "上传数据", "返回执行结果"})
      n190 = case shown="\"上传数据\"" w307 {
        tunnel: ["QnRtn=1" w309 "ExeRtn=1"] -> w306
        frame "返回请求应答", Default {
        }
        frame "上传数据" {
          n191 = Get Date/Time In Seconds() -> (seconds since 1Jan1904=w313:timestamp)
          n192 = Format Date/Time String(time format string (%c)="%Y%m%d%H%M%S" ("时间格式字符串(%c)"), seconds (now)=w313) -> (date/time string=w310:string)  [unwired: 1 in]
          n193 = Concatenate Strings("SystemTime=", w310) -> (w309:string)
        }
        frame "返回执行结果" {
        }
      }
    }
    frame "获取软件版本号" {
      (unwired) ""
      n194 = global read "全局1.vi" "枚举"() -> (w316:enum16{"返回请求应答", "上传数据", "返回执行结果"})
      n195 = case shown="\"上传数据\"" w316 {
        tunnel: ["QnRtn=1" w319 "ExeRtn=1"] -> w315
        frame "返回请求应答", Default {
        }
        frame "上传数据" {
          n196 = global read "全局1.vi" "版本信息"() -> (w318:string)
          n197 = Concatenate Strings("Version=", w318) -> (w319:string)
        }
        frame "返回执行结果" {
        }
      }
    }
    frame "获取仪器软件版本号" {
      (unwired) ""
      n198 = global read "全局1.vi" "枚举"() -> (w323:enum16{"返回请求应答", "上传数据", "返回执行结果"})
      n199 = case shown="\"上传数据\"" w323 {
        tunnel: ["QnRtn=1" w329 "ExeRtn=1"] -> w322
        frame "返回请求应答", Default {
        }
        frame "上传数据" {
          n200 = global read "全局1.vi" "固件版本"() -> (w328:T7)
          n201 = global read "全局 小时数据发送次数.vi" "小时数据发送次数"() -> (w326:i32)
          n202 = Cluster To Array(cluster=w328) -> (array=w327:string[])
          n203 = Index Array(array=w327, index=w326) -> (element=w325:string)
          n204 = Concatenate Strings("FirmwareVersion=", w325) -> (w329:string)
        }
        frame "返回执行结果" {
        }
      }
    }
    frame "提取实时数据间隔" {
      (unwired) ""
      n205 = global read "全局1.vi" "枚举"() -> (w333:enum16{"返回请求应答", "上传数据", "返回执行结果"})
      n206 = case shown="\"上传数据\"" w333 {
        tunnel: ["QnRtn=1" w337 "ExeRtn=1"] -> w332
        frame "返回请求应答", Default {
        }
        frame "上传数据" {
          n207 = global read "实时数据发送间隔全局.vi" "实时数据发送间隔"() -> (w336:u32)
          n208 = Number To Decimal String(number=w336) -> (decimal integer string=w335:string)  [unwired: 1 in]
          n209 = Concatenate Strings("RtdInterval=", w335) -> (w337:string)
        }
        frame "返回执行结果" {
        }
      }
    }
    frame "实时数据" {
      # "包含质控数据主动上传"
      n210 = global read "全局 实时数据参数.vi" "实时数据参数"() -> (w342:string)
      n211 = case shown="\"集成干预测试\"" w342 {
        tunnel: [w346 w371 w396 w427 w451 w472] -> w343
        tunnel: w341 -> [w345 w370 w395 w425 w449 w470]
        tunnel: w340 -> [w344 w369 w394 w424 w448 w469]
        frame "水样测试", Default {
          n212 = global read "全局1.vi" "枚举"() -> (w347:enum16{"返回请求应答", "上传数据", "返回执行结果"})
          n213 = case shown="\"上传数据\"" w347 {
            tunnel: ["QnRtn=1" w365 "ExeRtn=1"] -> w346
            tunnel: w345 -> [_ w351 _]
            tunnel: w344 -> [_ w349 _]
            frame "返回请求应答", Default {
            }
            frame "上传数据" {
              n214 = call "数据发送组合-20200825 (子VI).vi"("枚举"=T4."实时数据", "插值后的数组元素"=w351) -> ("字符串"=w352:string)  [unwired: 9 in]
              n215 = global read "全局 小时数据发送次数.vi" "小时数据发送次数"() -> (w363:i32)
              n216 = Index Array(array=w349, index (row)=w363) -> (element=w362:string[])  [unwired: 1 in]
              n217 = Index Array(array=w362, index=0 ("索引")) -> (element=w360:string)
              n218 = call "规范时间戳.vi"("字符串"=w360) -> ("result string"=w358:string)  [unwired: 10 in]
              n219 = Empty String/Path?(string/path=w352) -> (empty?=w364:bool)
              n220 = Format Into String(format string="DataTime=%s;", w358) -> (resulting string=w357:string)  [unwired: 2 in, 1 out]
              n221 = Concatenate Strings(w357, w352) -> (w354:string)
              n222 = String Length(string=w354) -> (length=w356:i32)
              n223 = Decrement(x=w356) -> (x-1=w355:i32)
              n224 = String Subset(string=w354, length (rest)=w355) -> (substring=w353:string)  [unwired: 1 in]
              n225 = case shown="假" w364 {
                tunnel: [w366 ""] -> w365
                tunnel: w353 -> [w366 _]
                frame False {
                }
                frame True {
                }
              }
            }
            frame "返回执行结果" {
            }
          }
        }
        frame "平行样测试" {
          n226 = global read "全局1.vi" "枚举"() -> (w372:enum16{"返回请求应答", "上传数据", "返回执行结果"})
          n227 = case shown="\"上传数据\"" w372 {
            tunnel: ["QnRtn=1" w384 "ExeRtn=1"] -> w371
            tunnel: w369 -> [_ w378 _]
            tunnel: w370 -> [_ w375 _]
            frame "返回请求应答", Default {
            }
            frame "上传数据" {
              # "CODMn"
              n228 = call "数据发送组合-20200825 (子VI).vi"("枚举"=T4."平行样测试", "插值后的数组元素"=w375) -> ("字符串"=w374:string)  [unwired: 9 in]
              n229 = global read "全局 小时数据发送次数.vi" "小时数据发送次数"() -> (w377:i32)
              n230 = Index Array(array=w378, index (row)=w377) -> (element=w382:string[])  [unwired: 1 in]
              n231 = Index Array(array=w382, index=0 ("索引")) -> (element=w379:string)
              n232 = call "规范时间戳.vi"("字符串"=w379) -> ("result string"=w380:string)  [unwired: 10 in]
              n233 = Empty String/Path?(string/path=w379) -> (empty?=w383:bool)
              n234 = Format Into String(format string="DataTime=%s;%s" ("格式字符串"), w380, w374) -> (resulting string=w385:string)  [unwired: 2 in, 1 out]
              n235 = case shown="真" w383 {
                tunnel: [w389 ""] -> w384
                tunnel: w385 -> [w389 _]
                frame False {
                  n236 = global read "全局 小时数据发送次数.vi" "小时数据发送次数"() -> (w388:i32)
                  n237 = Increment(x=w388) -> (x+1=w387:i32)
                  n238 = global write "全局 小时数据发送次数.vi" "小时数据发送次数"(w387) -> ()
                }
                frame True {
                  n239 = global read "全局 小时数据发送次数.vi" "小时数据发送次数"() -> (w391:i32)
                  n240 = Increment(x=w391) -> (x+1=w390:i32)
                  n241 = global write "全局 小时数据发送次数.vi" "小时数据发送次数"(w390) -> ()
                }
              }
            }
            frame "返回执行结果" {
            }
          }
        }
        frame "集成干预测试" {
          n242 = global read "全局1.vi" "枚举"() -> (w397:enum16{"返回请求应答", "上传数据", "返回执行结果"})
          n243 = case shown="\"上传数据\"" w397 {
            tunnel: ["QnRtn=1" w410 "ExeRtn=1"] -> w396
            tunnel: w394 -> [_ w404 _]
            tunnel: w395 -> [_ w401 _]
            frame "返回请求应答", Default {
            }
            frame "上传数据" {
              # "CODMn"
              n244 = global read "全局 小时数据发送次数.vi" "小时数据发送次数"() -> (w403:i32)
              n245 = call "数据发送组合-20200825 (子VI).vi"("枚举"=T4."集成干预测试", "插值后的数组元素"=w401) -> ("字符串"=w400:string)  [unwired: 9 in]
              n246 = Index Array(array=w404, index (row)=w403) -> (element=w408:string[])  [unwired: 1 in]
              n247 = global read "断电保存全局.vi" "应用环境"() -> (w399:T8)
              n248 = Index Array(array=w408, index=0 ("索引")) -> (element=w405:string)
              n249 = case shown="\"GB212\", 默认" w399 {
                tunnel: [w414 w415] -> w406
                tunnel: w405 -> [w413 w416]
                frame "STD" {
                  n250 = call "规范时间戳.vi"("字符串"=w413) -> ("result string"=w414:string)  [unwired: 10 in]
                }
                frame "GB212", Default {
                  n251 = call "规范分钟数据时间戳.vi"("字符串"=w416) -> ("result string"=w415:string)  [unwired: 10 in]
                }
              }
              n252 = Empty String/Path?(string/path=w405) -> (empty?=w409:bool)
              n253 = Format Into String(format string="DataTime=%s;%s" ("格式字符串"), w406, w400) -> (resulting string=w411:string)  [unwired: 2 in, 1 out]
              n254 = case shown="假" w409 {
                tunnel: [w419 ""] -> w410
                tunnel: w411 -> [w419 _]
                frame False {
                  n255 = global read "全局 小时数据发送次数.vi" "小时数据发送次数"() -> (w418:i32)
                  n256 = Increment(x=w418) -> (x+1=w417:i32)
                  n257 = global write "全局 小时数据发送次数.vi" "小时数据发送次数"(w417) -> ()
                }
                frame True {
                  n258 = global read "全局 小时数据发送次数.vi" "小时数据发送次数"() -> (w421:i32)
                  n259 = Increment(x=w421) -> (x+1=w420:i32)
                  n260 = global write "全局 小时数据发送次数.vi" "小时数据发送次数"(w420) -> ()
                }
              }
            }
            frame "返回执行结果" {
            }
          }
        }
        frame "加标回收测试" {
          n261 = global read "全局1.vi" "枚举"() -> (w426:enum16{"返回请求应答", "上传数据", "返回执行结果"})
          n262 = case shown="\"上传数据\"" w426 {
            tunnel: ["QnRtn=1" w437 "ExeRtn=1"] -> w427
            tunnel: w424 -> [_ w432 _]
            tunnel: w425 -> [_ w434 _]
            frame "返回请求应答", Default {
            }
            frame "上传数据" {
              # "w01001-Check=63.0,w01001-WaterTime=20160801080000,w01001-Water=45.23,w01001-Chroma=1000,w01001-Volume=0.2,w01001-DVolume=200,w01003-Flag=N;"
              # "CODMn"
              n263 = global read "全局 小时数据发送次数.vi" "小时数据发送次数"() -> (w431:i32)
              n264 = call "加标回收数据组合 (子VI).vi"("小时数据发送次数"=w431, "数据"=w432, "污染物编码"="CODMn") -> ("datatime"=w430:string)  [unwired: 7 in, 1 out]
              n265 = call "规范时间戳.vi"("字符串"=w430) -> ("result string"=w439:string)  [unwired: 10 in]
              n266 = Empty String/Path?(string/path=w439) -> (empty?=w436:bool)
              n267 = call "数据发送组合-20200825 (子VI).vi"("枚举"=T4."加标回收测试", "插值后的数组元素"=w434) -> ("字符串"=w433:string)  [unwired: 9 in]
              n268 = Format Into String(format string="DataTime=%s;%s" ("格式字符串"), w439, w433) -> (resulting string=w438:string)  [unwired: 2 in, 1 out]
              n269 = case shown="真" w436 {
                tunnel: [w443 ""] -> w437
                tunnel: w438 -> [w443 _]
                frame False {
                  n270 = global read "全局 小时数据发送次数.vi" "小时数据发送次数"() -> (w442:i32)
                  n271 = Increment(x=w442) -> (x+1=w441:i32)
                  n272 = global write "全局 小时数据发送次数.vi" "小时数据发送次数"(w441) -> ()
                }
                frame True {
                  n273 = global read "全局 小时数据发送次数.vi" "小时数据发送次数"() -> (w445:i32)
                  n274 = Increment(x=w445) -> (x+1=w444:i32)
                  n275 = global write "全局 小时数据发送次数.vi" "小时数据发送次数"(w444) -> ()
                }
              }
            }
            frame "返回执行结果" {
            }
          }
        }
        frame "核查数据" {
          n276 = global read "全局1.vi" "枚举"() -> (w450:enum16{"返回请求应答", "上传数据", "返回执行结果"})
          n277 = case shown="\"上传数据\"" w450 {
            tunnel: ["QnRtn=1" w461 "ExeRtn=1"] -> w451
            tunnel: w449 -> [_ w454 _]
            tunnel: w448 -> [_ w453 _]
            frame "返回请求应答", Default {
            }
            frame "上传数据" {
              # "将非空数组的时间戳写入"
              n278 = global read "全局 小时数据发送次数.vi" "小时数据发送次数"() -> (w457:i32)
              n279 = Index Array(array=w453, index (row)=w457) -> (element=w460:string[])  [unwired: 1 in]
              n280 = call "数据发送组合-20200825 (子VI).vi"("枚举"=T4."核查数据", "插值后的数组元素"=w454) -> ("字符串"=w455:string)  [unwired: 9 in]
              n281 = Index Array(array=w460, index=0 ("索引")) -> (element=w459:string)
              n282 = call "规范分钟数据时间戳.vi"("字符串"=w459) -> ("result string"=w458:string)  [unwired: 10 in]
              n283 = Empty String/Path?(string/path=w458) -> (empty?=w463:bool)
              n284 = Format Into String(format string="DataTime=%s;%s" ("格式字符串"), w458, w455) -> (resulting string=w462:string)  [unwired: 2 in, 1 out]
              n285 = case shown="假" w463 {
                tunnel: [w466 ""] -> w461
                tunnel: w462 -> [w466 _]
                frame False {
                }
                frame True {
                }
              }
            }
            frame "返回执行结果" {
            }
          }
        }
        frame "空白测试", "跨度核查" {
          n286 = global read "全局1.vi" "枚举"() -> (w471:enum16{"返回请求应答", "上传数据", "返回执行结果"})
          n287 = case shown="\"上传数据\"" w471 {
            tunnel: ["QnRtn=1" w482 "ExeRtn=1"] -> w472
            tunnel: w470 -> [_ w476 _]
            tunnel: w469 -> [_ w474 _]
            frame "返回请求应答", Default {
            }
            frame "上传数据" {
              n288 = global read "全局 小时数据发送次数.vi" "小时数据发送次数"() -> (w480:i32)
              n289 = call "数据发送组合-20200825 (子VI).vi"("枚举"=T4."空白零点跨度数据", "插值后的数组元素"=w476) -> ("字符串"=w475:string)  [unwired: 9 in]
              n290 = Index Array(array=w474, index (row)=w480) -> (element=w486:string[])  [unwired: 1 in]
              n291 = Index Array(array=w486, index #1=0 ("索引"), index #2=3 ("索引"), index #3=7 ("索引")) -> (element #1=w479:string)  [unwired: 2 out]
              n292 = call "规范小时时间戳.vi"("字符串"=w479) -> ("result string"=w478:string)  [unwired: 10 in]
              n293 = Empty String/Path?(string/path=w478) -> (empty?=w483:bool)
              n294 = Format Into String(format string="DataTime=%s;%s" ("格式字符串"), w478, w475) -> (resulting string=w481:string)  [unwired: 2 in, 1 out]
              n295 = case shown="假" w483 {
                tunnel: [w489 ""] -> w482
                tunnel: w481 -> [w489 _]
                frame False {
                }
                frame True {
                }
              }
            }
            frame "返回执行结果" {
            }
          }
        }
      }
    }
    frame "小时数据" {
      # "发送小时数据"
      n296 = global read "全局1.vi" "枚举"() -> (w495:enum16{"返回请求应答", "上传数据", "返回执行结果"})
      n297 = case shown="\"上传数据\"" w495 {
        tunnel: ["QnRtn=1" w517 "ExeRtn=1"] -> w493
        tunnel: w494 -> [_ w505 _]
        tunnel: w492 -> [_ w502 _]
        frame "返回请求应答", Default {
          (unwired) 0 ("当前包数")
          n298 = global read "全局 数据数组大小.vi" "数据数组大小"() -> (w496:i32)
          n299 = global write "全局1.vi" "枚举"(enum16{"返回请求应答", "上传数据", "返回执行结果"}."上传数据" ("枚举")) -> ()
          n300 = Equal To 0?(x=w496) -> (x = 0?=w497:bool)
          n301 = case shown="真" w497 {
            frame False {
            }
            frame True {
              n302 = global read "全局 小时数据发送次数.vi" "小时数据发送次数"() -> (w501:i32)
              n303 = Increment(x=w501) -> (x+1=w500:i32)
              n304 = global write "全局 小时数据发送次数.vi" "小时数据发送次数"(w500) -> ()
            }
          }
        }
        frame "上传数据" {
          n305 = global read "全局 小时数据发送次数.vi" "小时数据发送次数"() -> (w516:i32)
          n306 = call "数据发送组合-20200825 (子VI).vi"("枚举"=enum16{"小时数据", "实时数据"}."小时数据", "插值后的数组元素"=w505) -> ("字符串"=w503:string)  [unwired: 9 in]
          n307 = Index Array(array=w502, index (row)=w516) -> (element=w515:string[])  [unwired: 1 in]
          n308 = Index Array(array=w515, index=0 ("索引")) -> (element=w513:string)
          n309 = call "规范小时时间戳.vi"("字符串"=w513) -> ("result string"=w510:string)  [unwired: 10 in]
          n310 = Empty String/Path?(string/path=w503) -> (empty?=w518:bool)
          n311 = Format Into String(format string="DataTime=%s;", w510) -> (resulting string=w512:string)  [unwired: 2 in, 1 out]
          n312 = Concatenate Strings(w512, w503) -> (w507:string)
          n313 = String Length(string=w507) -> (length=w509:i32)
          n314 = Decrement(x=w509) -> (x-1=w508:i32)
          n315 = String Subset(string=w507, length (rest)=w508) -> (substring=w506:string)  [unwired: 1 in]
          n316 = case shown="假" w518 {
            tunnel: [w519 ""] -> w517
            tunnel: w506 -> [w519 _]
            frame False {
            }
            frame True {
            }
          }
        }
        frame "返回执行结果" {
          (unwired) 0 ("当前包数")
          n317 = global write "全局1.vi" "枚举"(enum16{"返回请求应答", "上传数据", "返回执行结果"}."返回请求应答" ("枚举")) -> ()
        }
      }
    }
    frame "剖面数据" {
      # "{\"data\":[{\"time\":\"21-06-08 01:08:00\",\"w01010Value\":23,\"w01001Value\":7,\"w01009Value\":6,\"w01014Value\":22,\"w01003Value\":100,\"depth\":0.5,\"row\":3},{\"time\":\"21-06-08 01:08:00\",\"w01010Value\":22,\"w01001Value\":8,\"w01009Value\":7,\"w01014Value\":25,\"w01003Value\":96,\"depth\":0.8,\"row\":3},{\"time\":\"21-06-08 01:08:00\",\"w01010Value\":21,\"w01001Value\":7,\"w01009Value\":7,\"w01014Value\":24,\"w01003Value\":95,\"depth\":1,\"row\":3}]}"
      # "发送剖面数据"
      n318 = global read "全局1.vi" "枚举"() -> (w523:enum16{"返回请求应答", "上传数据", "返回执行结果"})
      n319 = case shown="\"上传数据\"" w523 {
        tunnel: ["QnRtn=1" w534 "ExeRtn=1"] -> w524
        frame "返回请求应答", Default {
          (unwired) 0 ("当前包数")
          n320 = global read "全局 数据数组大小.vi" "数据数组大小"() -> (w525:i32)
          n321 = global write "全局1.vi" "枚举"(enum16{"返回请求应答", "上传数据", "返回执行结果"}."上传数据" ("枚举")) -> ()
          n322 = Equal To 0?(x=w525) -> (x = 0?=w526:bool)
          n323 = case shown="真" w526 {
            frame False {
            }
            frame True {
              n324 = global read "全局 小时数据发送次数.vi" "小时数据发送次数"() -> (w530:i32)
              n325 = Increment(x=w530) -> (x+1=w529:i32)
              n326 = global write "全局 小时数据发送次数.vi" "小时数据发送次数"(w529) -> ()
            }
          }
        }
        frame "上传数据" {
          n327 = global read "断电保存全局.vi" "数据发送协议"() -> (w533:enum16{"2005-212协议", "2017-212协议"})
          n328 = case shown="\"2017-212协议\", 默认" w533 {
            tunnel: ["" ("编码输出") w555] -> w532
            tunnel: [_ w551] -> w531
            frame "2005-212协议" {
            }
            frame "2017-212协议", Default {
              w545 = 0 ("索引 (行)")
              (unwired) "w01010" ("污染物编码")
              (unwired) "w01016" ("污染物编码")
              (unwired) "w01003" ("污染物编码")
              (unwired) "w01014" ("污染物编码")
              # "时间,测量模式,数据类型,数据标识,层数,Temp,SpCond,Cond,Sal,TDS,pH,pHmV,ORP,ODO%,ODOmg/L,Turb,Chla,Depth,"
              n329 = global read "全局 小时数据发送次数.vi" "小时数据发送次数"() -> (w554:i32)
              n330 = global read "全局 所有参数.vi" "剖面多参数"() -> (w542:string[][])
              n331 = global read "全局 数据数组大小.vi" "分包标准"() -> (w553:i32)
              n332 = global read "全局 所有参数.vi" "columns"() -> (w552:string[])
              n333 = Array Subset(array=w542, index (row)=w554, length (row)=w553) -> (w551:string[][])  [unwired: 2 in]
              n334 = Array Subset(array=w542, index (row)=0 ("索引"), length (row)=1 ("长度")) -> (w540:string[][])  [unwired: 2 in]
              n335 = call "新剖面数据组合.vi"("columns"=w552, "剖面数据"=w551) -> ("结果字符串"=w549:string)  [unwired: 9 in]
              n336 = Index Array(array=w540, index (row) #1=w545, index (col) #1=0 ("索引 (行)"), index (row) #2=w545, index (col) #2=1 ("索引 (列)"), index (row) #3=w545, index (col) #3=2 ("索引 (列)")) -> (element #1=w538:string, element #2=w544:string, element #3=w543:string)
              n337 = call "规范小时时间戳.vi"("字符串"=w538) -> ("result string"=w537:string)  [unwired: 10 in]
              n338 = Empty String/Path?(string/path=w549) -> (empty?=w556:bool)
              n339 = Format Into String(format string="DataTime=%s;total=%s;waterdepth=%s;data=%s", w537, w544, w543, w549) -> (resulting string=w548:string)  [unwired: 2 in, 1 out]
              n340 = case shown="真" w556 {
                tunnel: [w558 ""] -> w555
                tunnel: w548 -> [w558 _]
                frame False {
                }
                frame True {
                }
              }
            }
          }
          n341 = Empty String/Path?(string/path=w532) -> (empty?=w535:bool)
          n342 = case shown="假" w535 {
            tunnel: [w565 ""] -> w534
            tunnel: w532 -> [w565 _]
            tunnel: w531 -> [w564 w566]
            frame False {
              n343 = Array Size(array=w564) -> (size(s)=w563:i32[])
              n344 = global read "全局 小时数据发送次数.vi" "小时数据发送次数"() -> (w561:i32)
              n345 = Index Array(array=w563) -> (element=w562:i32)  [unwired: 1 in]
              n346 = Add(x=w562, y=w561) -> (x+y=w560:i32)
              n347 = global write "全局 小时数据发送次数.vi" "小时数据发送次数"(w560) -> ()
            }
            frame True {
              n348 = Array Size(array=w566) -> (size(s)=w570:i32[])
              n349 = global read "全局 小时数据发送次数.vi" "小时数据发送次数"() -> (w568:i32)
              n350 = Index Array(array=w570) -> (element=w569:i32)  [unwired: 1 in]
              n351 = Add(x=w569, y=w568) -> (x+y=w567:i32)
              n352 = global write "全局 小时数据发送次数.vi" "小时数据发送次数"(w567) -> ()
            }
          }
        }
        frame "返回执行结果" {
          (unwired) 0 ("当前包数")
          n353 = global write "全局1.vi" "枚举"(enum16{"返回请求应答", "上传数据", "返回执行结果"}."返回请求应答" ("枚举")) -> ()
        }
      }
    }
    frame "剖面多参数H" {
      # "发送小时数据"
      n354 = global read "全局1.vi" "枚举"() -> (w574:enum16{"返回请求应答", "上传数据", "返回执行结果"})
      n355 = case shown="\"上传数据\"" w574 {
        tunnel: ["QnRtn=1" w584 "ExeRtn=1"] -> w575
        frame "返回请求应答", Default {
          (unwired) 0 ("当前包数")
          n356 = global read "全局 数据数组大小.vi" "数据数组大小"() -> (w576:i32)
          n357 = global write "全局1.vi" "枚举"(enum16{"返回请求应答", "上传数据", "返回执行结果"}."上传数据" ("枚举")) -> ()
          n358 = Equal To 0?(x=w576) -> (x = 0?=w577:bool)
          n359 = case shown="真" w577 {
            frame False {
            }
            frame True {
              n360 = global read "全局 小时数据发送次数.vi" "小时数据发送次数"() -> (w581:i32)
              n361 = Increment(x=w581) -> (x+1=w580:i32)
              n362 = global write "全局 小时数据发送次数.vi" "小时数据发送次数"(w580) -> ()
            }
          }
        }
        frame "上传数据" {
          n363 = global read "断电保存全局.vi" "数据发送协议"() -> (w583:enum16{"2005-212协议", "2017-212协议"})
          n364 = case shown="\"2017-212协议\", 默认" w583 {
            tunnel: ["" ("编码输出") w590] -> w582
            frame "2005-212协议" {
            }
            frame "2017-212协议", Default {
              (unwired) "w01010" ("污染物编码")
              (unwired) "w01016" ("污染物编码")
              (unwired) "w01003" ("污染物编码")
              (unwired) "w01009" ("污染物编码")
              (unwired) "w01001" ("污染物编码")
              (unwired) "w01014" ("污染物编码")
              (unwired) "w01100" ("污染物编码")
              # "时间,测量模式,数据类型,数据标识,层数,Temp,SpCond,Cond,Sal,TDS,pH,pHmV,ORP,ODO%,ODOmg/L,Turb,Chla,Depth,"
              n365 = global read "全局 小时数据发送次数.vi" "小时数据发送次数"() -> (w608:i32)
              n366 = global read "全局 所有参数.vi" "剖面多参数"() -> (w611:string[][])
              n367 = Index Array(array=w611, index (row)=w608) -> (element=w609:string[])  [unwired: 1 in]
              n368 = Index Array(array=w609, index #1=0 ("索引")) -> (element #1=w593:string, element #3=w607:string, element #4=w606:string, element #5=w605:string, element #6=w604:string, element #7=w603:string, element #11=w601:string, element #13=w600:string, element #15=w599:string, element #16=w598:string, element #17=w597:string, element #18=w587:string)  [unwired: 17 in, 6 out]
              n369 = call "规范小时时间戳.vi"("字符串"=w593) -> ("result string"=w594:string)  [unwired: 10 in]
              n370 = Build Array(w604, w603, w601, w600, w599, w598, w597, w587) -> (w602:string[])
              n371 = call "剖面多参数组合(子VI).vi"("数据类型实时小时"="-Avg=", "数据值"=w602, "层数"=w605, "数据标识"=w606, "数据类型"=w607) -> ("编码输出"=w589:string)  [unwired: 6 in]
              n372 = Format Into String(format string="DataTime=%s;", w594) -> (resulting string=w595:string)  [unwired: 2 in, 1 out]
              n373 = Empty String/Path?(string/path=w589) -> (empty?=w592:bool)
              n374 = Concatenate Strings(w595, w589) -> (w591:string)
              n375 = case shown="真" w592 {
                tunnel: [w612 ""] -> w590
                tunnel: w591 -> [w612 _]
                frame False {
                }
                frame True {
                }
              }
            }
          }
          n376 = Empty String/Path?(string/path=w582) -> (empty?=w585:bool)
          n377 = case shown="假" w585 {
            tunnel: [w616 ""] -> w584
            tunnel: w582 -> [w616 _]
            frame False {
              n378 = global read "全局 小时数据发送次数.vi" "小时数据发送次数"() -> (w615:i32)
              n379 = Increment(x=w615) -> (x+1=w614:i32)
              n380 = global write "全局 小时数据发送次数.vi" "小时数据发送次数"(w614) -> ()
            }
            frame True {
              n381 = global read "全局 小时数据发送次数.vi" "小时数据发送次数"() -> (w618:i32)
              n382 = Increment(x=w618) -> (x+1=w617:i32)
              n383 = global write "全局 小时数据发送次数.vi" "小时数据发送次数"(w617) -> ()
            }
          }
        }
        frame "返回执行结果" {
          (unwired) 0 ("当前包数")
          n384 = global write "全局1.vi" "枚举"(enum16{"返回请求应答", "上传数据", "返回执行结果"}."返回请求应答" ("枚举")) -> ()
        }
      }
    }
    frame "剖面多参数S" {
      # "发送实时数据"
      n385 = global read "全局1.vi" "枚举"() -> (w622:enum16{"返回请求应答", "上传数据", "返回执行结果"})
      n386 = case shown="\"上传数据\"" w622 {
        tunnel: ["QnRtn=1" w632 "ExeRtn=1"] -> w623
        frame "返回请求应答", Default {
          (unwired) 0 ("当前包数")
          n387 = global read "全局 数据数组大小.vi" "数据数组大小"() -> (w624:i32)
          n388 = global write "全局1.vi" "枚举"(enum16{"返回请求应答", "上传数据", "返回执行结果"}."上传数据" ("枚举")) -> ()
          n389 = Equal To 0?(x=w624) -> (x = 0?=w625:bool)
          n390 = case shown="真" w625 {
            frame False {
            }
            frame True {
              n391 = global read "全局 小时数据发送次数.vi" "小时数据发送次数"() -> (w629:i32)
              n392 = Increment(x=w629) -> (x+1=w628:i32)
              n393 = global write "全局 小时数据发送次数.vi" "小时数据发送次数"(w628) -> ()
            }
          }
        }
        frame "上传数据" {
          n394 = global read "断电保存全局.vi" "数据发送协议"() -> (w631:enum16{"2005-212协议", "2017-212协议"})
          n395 = case shown="\"2017-212协议\", 默认" w631 {
            tunnel: ["" ("编码输出") w640] -> w630
            frame "2005-212协议" {
            }
            frame "2017-212协议", Default {
              (unwired) "w01010" ("污染物编码")
              (unwired) "w01016" ("污染物编码")
              (unwired) "w01003" ("污染物编码")
              (unwired) "w01009" ("污染物编码")
              (unwired) "w01001" ("污染物编码")
              (unwired) "w01014" ("污染物编码")
              (unwired) "w01100" ("污染物编码")
              # "时间,测量模式,数据类型,数据标识,层数,Temp,SpCond,Cond,Sal,TDS,pH,pHmV,ORP,ODO%,ODOmg/L,Turb,Chla,Depth,"
              n396 = global read "全局 小时数据发送次数.vi" "小时数据发送次数"() -> (w656:i32)
              n397 = global read "全局 所有参数.vi" "剖面多参数"() -> (w659:string[][])
              n398 = Index Array(array=w659, index (row)=w656) -> (element=w657:string[])  [unwired: 1 in]
              n399 = Index Array(array=w657, index #1=0 ("索引")) -> (element #1=w637:string, element #3=w655:string, element #4=w654:string, element #5=w653:string, element #6=w652:string, element #7=w651:string, element #11=w649:string, element #13=w648:string, element #15=w647:string, element #16=w646:string, element #17=w645:string, element #18=w635:string)  [unwired: 17 in, 6 out]
              n400 = call "规范时间戳.vi"("字符串"=w637) -> ("result string"=w636:string)  [unwired: 10 in]
              n401 = Build Array(w652, w651, w649, w648, w647, w646, w645, w635) -> (w650:string[])
              n402 = call "剖面多参数组合(子VI).vi"("数据类型实时小时"="-Rtd=", "数据值"=w650, "层数"=w653, "数据标识"=w654, "数据类型"=w655) -> ("编码输出"=w639:string)  [unwired: 6 in]
              n403 = Format Into String(format string="DataTime=%s;", w636) -> (resulting string=w643:string)  [unwired: 2 in, 1 out]
              n404 = Empty String/Path?(string/path=w639) -> (empty?=w642:bool)
              n405 = Concatenate Strings(w643, w639) -> (w641:string)
              n406 = case shown="假" w642 {
                tunnel: [w660 ""] -> w640
                tunnel: w641 -> [w660 _]
                frame False {
                }
                frame True {
                }
              }
            }
          }
          n407 = Empty String/Path?(string/path=w630) -> (empty?=w633:bool)
          n408 = case shown="假" w633 {
            tunnel: [w664 ""] -> w632
            tunnel: w630 -> [w664 _]
            frame False {
              n409 = global read "全局 小时数据发送次数.vi" "小时数据发送次数"() -> (w663:i32)
              n410 = Increment(x=w663) -> (x+1=w662:i32)
              n411 = global write "全局 小时数据发送次数.vi" "小时数据发送次数"(w662) -> ()
            }
            frame True {
              n412 = global read "全局 小时数据发送次数.vi" "小时数据发送次数"() -> (w666:i32)
              n413 = Increment(x=w666) -> (x+1=w665:i32)
              n414 = global write "全局 小时数据发送次数.vi" "小时数据发送次数"(w665) -> ()
            }
          }
        }
        frame "返回执行结果" {
          (unwired) 0 ("当前包数")
          n415 = global write "全局1.vi" "枚举"(enum16{"返回请求应答", "上传数据", "返回执行结果"}."返回请求应答" ("枚举")) -> ()
        }
      }
    }
    frame "提取小时数据" {
      # "发送小时数据"
      n416 = global read "全局 小时数据发送次数.vi" "小时数据发送次数"() -> (w672:i32)
      n417 = Index Array(array=w674, index (row)=w672) -> (element=w671:string[])  [unwired: 1 in]
      n418 = global read "全局1.vi" "枚举"() -> (w673:enum16{"返回请求应答", "上传数据", "返回执行结果"})
      n419 = case shown="\"上传数据\"" w673 {
        tunnel: ["QnRtn=1" w689 "ExeRtn=1"] -> w675
        tunnel: w671 -> [_ w691 _]
        tunnel: w670 -> [_ w681 _]
        frame "返回请求应答", Default {
          n420 = global read "全局 数据数组大小.vi" "数据数组大小"() -> (w676:i32)
          n421 = Equal To 0?(x=w676) -> (x = 0?=w677:bool)
          n422 = case shown="真" w677 {
            frame False {
            }
            frame True {
              n423 = global read "全局 小时数据发送次数.vi" "小时数据发送次数"() -> (w680:i32)
              n424 = Increment(x=w680) -> (x+1=w679:i32)
              n425 = global write "全局 小时数据发送次数.vi" "小时数据发送次数"(w679) -> ()
            }
          }
        }
        frame "上传数据" {
          n426 = Index Array(array=w691, index #2=1 ("索引")) -> (element #1=w684:string)  [unwired: 1 in, 1 out]
          n427 = call "规范小时时间戳.vi"("字符串"=w684) -> ("result string"=w685:string)  [unwired: 10 in]
          n428 = call "数据发送组合-20200825 (子VI).vi"("枚举"=T4."提取小时数据", "插值后的数组元素"=w681) -> ("字符串"=w682:string)  [unwired: 9 in]
          n429 = Format Into String(format string="DataTime=%s;", w685) -> (resulting string=w688:string)  [unwired: 2 in, 1 out]
          n430 = Empty String/Path?(string/path=w682) -> (empty?=w690:bool)
          n431 = Concatenate Strings(w688, w682) -> (w686:string)
          n432 = case shown="假" w690 {
            tunnel: [w695 ""] -> w689
            tunnel: w686 -> [w695 _]
            frame False {
              n433 = global read "全局 小时数据发送次数.vi" "小时数据发送次数"() -> (w694:i32)
              n434 = Increment(x=w694) -> (x+1=w693:i32)
              n435 = global write "全局 小时数据发送次数.vi" "小时数据发送次数"(w693) -> ()
            }
            frame True {
              n436 = global read "全局 小时数据发送次数.vi" "小时数据发送次数"() -> (w697:i32)
              n437 = Increment(x=w697) -> (x+1=w696:i32)
              n438 = global write "全局 小时数据发送次数.vi" "小时数据发送次数"(w696) -> ()
            }
          }
        }
        frame "返回执行结果" {
        }
      }
    }
    frame "提取实时数据" {
      # "提取实时数据"
      n439 = global read "全局 小时数据发送次数.vi" "小时数据发送次数"() -> (w702:i32)
      n440 = Index Array(array=w705, index (row)=w702) -> (element=w701:string[])  [unwired: 1 in]
      n441 = global read "全局1.vi" "枚举"() -> (w703:enum16{"返回请求应答", "上传数据", "返回执行结果"})
      n442 = case shown="\"上传数据\"" w703 {
        tunnel: ["QnRtn=1" w714 "ExeRtn=1"] -> w704
        tunnel: w701 -> [_ w720 _]
        tunnel: w700 -> [_ w712 _]
        frame "返回请求应答", Default {
          n443 = global read "全局 数据数组大小.vi" "数据数组大小"() -> (w706:i32)
          n444 = Equal To 0?(x=w706) -> (x = 0?=w707:bool)
          n445 = case shown="真" w707 {
            frame False {
            }
            frame True {
              n446 = global read "全局 小时数据发送次数.vi" "小时数据发送次数"() -> (w710:i32)
              n447 = Increment(x=w710) -> (x+1=w709:i32)
              n448 = global write "全局 小时数据发送次数.vi" "小时数据发送次数"(w709) -> ()
            }
          }
        }
        frame "上传数据" {
          n449 = Index Array(array=w720, index #1=0 ("索引"), index #2=3 ("索引"), index #3=5 ("索引")) -> (element #1=w718:string)  [unwired: 2 out]
          n450 = call "规范时间戳.vi"("字符串"=w718) -> ("result string"=w717:string)  [unwired: 10 in]
          n451 = call "数据发送组合-20200825 (子VI).vi"("枚举"=T4."提取实时数据", "插值后的数组元素"=w712) -> ("字符串"=w711:string)  [unwired: 9 in]
          n452 = Empty String/Path?(string/path=w717) -> (empty?=w716:bool)
          n453 = Format Into String(format string="DataTime=%s;%s" ("格式字符串"), w717, w711) -> (resulting string=w715:string)  [unwired: 2 in, 1 out]
          n454 = case shown="真" w716 {
            tunnel: [w724 ""] -> w714
            tunnel: w715 -> [w724 _]
            frame False {
              n455 = global read "全局 小时数据发送次数.vi" "小时数据发送次数"() -> (w726:i32)
              n456 = Increment(x=w726) -> (x+1=w725:i32)
              n457 = global write "全局 小时数据发送次数.vi" "小时数据发送次数"(w725) -> ()
            }
            frame True {
              n458 = global read "全局 小时数据发送次数.vi" "小时数据发送次数"() -> (w728:i32)
              n459 = Increment(x=w728) -> (x+1=w727:i32)
              n460 = global write "全局 小时数据发送次数.vi" "小时数据发送次数"(w727) -> ()
            }
          }
        }
        frame "返回执行结果" {
        }
      }
    }
    frame "核查数据" {
      # "提取标样核查数据"
      n461 = global read "全局 小时数据发送次数.vi" "小时数据发送次数"() -> (w734:i32)
      n462 = Index Array(array=w731, index (row)=w734) -> (element=w733:string[])  [unwired: 1 in]
      n463 = global read "全局1.vi" "枚举"() -> (w735:enum16{"返回请求应答", "上传数据", "返回执行结果"})
      n464 = case shown="\"上传数据\"" w735 {
        tunnel: ["QnRtn=1" w747 "ExeRtn=1"] -> w736
        tunnel: w733 -> [_ w753 _]
        tunnel: w732 -> [_ w743 _]
        frame "返回请求应答", Default {
          n465 = global read "全局 数据数组大小.vi" "数据数组大小"() -> (w738:i32)
          n466 = Equal To 0?(x=w738) -> (x = 0?=w737:bool)
          n467 = case shown="真" w737 {
            frame False {
            }
            frame True {
              n468 = global read "全局 小时数据发送次数.vi" "小时数据发送次数"() -> (w741:i32)
              n469 = Increment(x=w741) -> (x+1=w740:i32)
              n470 = global write "全局 小时数据发送次数.vi" "小时数据发送次数"(w740) -> ()
            }
          }
        }
        frame "上传数据" {
          # "将非空数组的时间戳写入"
          n471 = Index Array(array=w753, index #1=0 ("索引"), index #2=3 ("索引"), index #3=6 ("索引")) -> (element #1=w746:string)  [unwired: 2 out]
          n472 = call "数据发送组合-20200825 (子VI).vi"("枚举"=T4."核查数据", "插值后的数组元素"=w743) -> ("字符串"=w742:string)  [unwired: 9 in]
          n473 = call "规范时间戳.vi"("字符串"=w746) -> ("result string"=w745:string)  [unwired: 10 in]
          n474 = Empty String/Path?(string/path=w745) -> (empty?=w749:bool)
          n475 = Format Into String(format string="DataTime=%s;%s" ("格式字符串"), w745, w742) -> (resulting string=w748:string)  [unwired: 2 in, 1 out]
          n476 = case shown="假" w749 {
            tunnel: [w757 ""] -> w747
            tunnel: w748 -> [w757 _]
            frame False {
              n477 = global read "全局 小时数据发送次数.vi" "小时数据发送次数"() -> (w756:i32)
              n478 = Increment(x=w756) -> (x+1=w755:i32)
              n479 = global write "全局 小时数据发送次数.vi" "小时数据发送次数"(w755) -> ()
            }
            frame True {
              n480 = global read "全局 小时数据发送次数.vi" "小时数据发送次数"() -> (w759:i32)
              n481 = Increment(x=w759) -> (x+1=w758:i32)
              n482 = global write "全局 小时数据发送次数.vi" "小时数据发送次数"(w758) -> ()
            }
          }
        }
        frame "返回执行结果" {
        }
      }
    }
    frame "空白测试", "跨度核查", "零点核查" {
      # "提取空白测试数据/零点核查数据/跨度核查数据"
      n483 = global read "全局 小时数据发送次数.vi" "小时数据发送次数"() -> (w765:i32)
      n484 = Index Array(array=w762, index (row)=w765) -> (element=w764:string[])  [unwired: 1 in]
      n485 = global read "全局1.vi" "枚举"() -> (w766:enum16{"返回请求应答", "上传数据", "返回执行结果"})
      n486 = case shown="\"上传数据\"" w766 {
        tunnel: ["QnRtn=1" w778 "ExeRtn=1"] -> w767
        tunnel: w764 -> [_ w783 _]
        tunnel: w763 -> [_ w774 _]
        frame "返回请求应答", Default {
          (unwired) 0 ("当前包数")
          n487 = global read "全局 数据数组大小.vi" "数据数组大小"() -> (w769:i32)
          n488 = Equal To 0?(x=w769) -> (x = 0?=w768:bool)
          n489 = case shown="真" w768 {
            frame False {
            }
            frame True {
              n490 = global read "全局 小时数据发送次数.vi" "小时数据发送次数"() -> (w772:i32)
              n491 = Increment(x=w772) -> (x+1=w771:i32)
              n492 = global write "全局 小时数据发送次数.vi" "小时数据发送次数"(w771) -> ()
            }
          }
        }
        frame "上传数据" {
          # "将非空数组的时间戳写入"
          n493 = Index Array(array=w783, index #1=0 ("索引"), index #2=3 ("索引")) -> (element #1=w777:string)  [unwired: 1 out]
          n494 = call "数据发送组合-20200825 (子VI).vi"("枚举"=T4."空白零点跨度数据", "插值后的数组元素"=w774) -> ("字符串"=w773:string)  [unwired: 9 in]
          n495 = call "规范时间戳.vi"("字符串"=w777) -> ("result string"=w776:string)  [unwired: 10 in]
          n496 = Empty String/Path?(string/path=w776) -> (empty?=w780:bool)
          n497 = Format Into String(format string="DataTime=%s;%s" ("格式字符串"), w776, w773) -> (resulting string=w779:string)  [unwired: 2 in, 1 out]
          n498 = case shown="假" w780 {
            tunnel: [w787 ""] -> w778
            tunnel: w779 -> [w787 _]
            frame False {
              n499 = global read "全局 小时数据发送次数.vi" "小时数据发送次数"() -> (w786:i32)
              n500 = Increment(x=w786) -> (x+1=w785:i32)
              n501 = global write "全局 小时数据发送次数.vi" "小时数据发送次数"(w785) -> ()
            }
            frame True {
              n502 = global read "全局 小时数据发送次数.vi" "小时数据发送次数"() -> (w789:i32)
              n503 = Increment(x=w789) -> (x+1=w788:i32)
              n504 = global write "全局 小时数据发送次数.vi" "小时数据发送次数"(w788) -> ()
            }
          }
        }
        frame "返回执行结果" {
        }
      }
    }
    frame "提取加标回收" {
      # "提取加标回收数据"
      n505 = global read "全局1.vi" "枚举"() -> (w795:enum16{"返回请求应答", "上传数据", "返回执行结果"})
      n506 = case shown="\"上传数据\"" w795 {
        tunnel: ["QnRtn=1" w807 "ExeRtn=1"] -> w793
        tunnel: w794 -> [_ w809 _]
        tunnel: w792 -> [_ w801 _]
        frame "返回请求应答", Default {
          n507 = global read "全局 数据数组大小.vi" "数据数组大小"() -> (w796:i32)
          n508 = Equal To 0?(x=w796) -> (x = 0?=w797:bool)
          n509 = case shown="真" w797 {
            frame False {
            }
            frame True {
              n510 = global read "全局 小时数据发送次数.vi" "小时数据发送次数"() -> (w800:i32)
              n511 = Increment(x=w800) -> (x+1=w799:i32)
              n512 = global write "全局 小时数据发送次数.vi" "小时数据发送次数"(w799) -> ()
            }
          }
        }
        frame "上传数据" {
          # "w01001-Check=63.0,w01001-WaterTime=20160801080000,w01001-Water=45.23,w01001-Chroma=1000,w01001-Volume=0.2,w01001-DVolume=200,w01003-Flag=N;"
          # "CODMn"
          n513 = global read "全局 小时数据发送次数.vi" "小时数据发送次数"() -> (w804:i32)
          n514 = call "数据发送组合-20200825 (子VI).vi"("枚举"=T4."加标回收测试", "插值后的数组元素"=w801) -> ("字符串"=w802:string)  [unwired: 9 in]
          n515 = call "加标回收数据组合 (子VI).vi"("小时数据发送次数"=w804, "数据"=w809, "污染物编码"="w01019") -> ("datatime"=w811:string)  [unwired: 7 in, 1 out]
          n516 = call "规范时间戳.vi"("字符串"=w811) -> ("result string"=w810:string)  [unwired: 10 in]
          n517 = Empty String/Path?(string/path=w810) -> (empty?=w806:bool)
          n518 = Format Into String(format string="DataTime=%s;%s" ("格式字符串"), w810, w802) -> (resulting string=w808:string)  [unwired: 2 in, 1 out]
          n519 = case shown="真" w806 {
            tunnel: [w815 ""] -> w807
            tunnel: w808 -> [w815 _]
            frame False {
              n520 = global read "全局 小时数据发送次数.vi" "小时数据发送次数"() -> (w814:i32)
              n521 = Increment(x=w814) -> (x+1=w813:i32)
              n522 = global write "全局 小时数据发送次数.vi" "小时数据发送次数"(w813) -> ()
            }
            frame True {
              n523 = global read "全局 小时数据发送次数.vi" "小时数据发送次数"() -> (w817:i32)
              n524 = Increment(x=w817) -> (x+1=w816:i32)
              n525 = global write "全局 小时数据发送次数.vi" "小时数据发送次数"(w816) -> ()
            }
          }
        }
        frame "返回执行结果" {
        }
      }
    }
    frame "提取平行样" {
      # "提取平行样数据"
      n526 = global read "全局1.vi" "枚举"() -> (w823:enum16{"返回请求应答", "上传数据", "返回执行结果"})
      n527 = case shown="\"上传数据\"" w823 {
        tunnel: ["QnRtn=1" w839 "ExeRtn=1"] -> w822
        tunnel: w821 -> [_ w833 _]
        tunnel: w820 -> [_ w829 _]
        frame "返回请求应答", Default {
          n528 = global read "全局 数据数组大小.vi" "数据数组大小"() -> (w824:i32)
          n529 = Equal To 0?(x=w824) -> (x = 0?=w825:bool)
          n530 = case shown="真" w825 {
            frame False {
            }
            frame True {
              n531 = global read "全局 小时数据发送次数.vi" "小时数据发送次数"() -> (w828:i32)
              n532 = Increment(x=w828) -> (x+1=w827:i32)
              n533 = global write "全局 小时数据发送次数.vi" "小时数据发送次数"(w827) -> ()
            }
          }
        }
        frame "上传数据" {
          # "CODMn"
          n534 = global read "全局 小时数据发送次数.vi" "小时数据发送次数"() -> (w832:i32)
          n535 = call "数据发送组合-20200825 (子VI).vi"("枚举"=T4."平行样测试", "插值后的数组元素"=w829) -> ("字符串"=w830:string)  [unwired: 9 in]
          n536 = Index Array(array=w833, index (row)=w832) -> (element=w837:string[])  [unwired: 1 in]
          n537 = Index Array(array=w837, index=0 ("索引")) -> (element=w834:string)
          n538 = call "规范时间戳.vi"("字符串"=w834) -> ("result string"=w835:string)  [unwired: 10 in]
          n539 = Empty String/Path?(string/path=w834) -> (empty?=w838:bool)
          n540 = Format Into String(format string="DataTime=%s;%s" ("格式字符串"), w835, w830) -> (resulting string=w840:string)  [unwired: 2 in, 1 out]
          n541 = case shown="真" w838 {
            tunnel: [w844 ""] -> w839
            tunnel: w840 -> [w844 _]
            frame False {
              n542 = global read "全局 小时数据发送次数.vi" "小时数据发送次数"() -> (w843:i32)
              n543 = Increment(x=w843) -> (x+1=w842:i32)
              n544 = global write "全局 小时数据发送次数.vi" "小时数据发送次数"(w842) -> ()
            }
            frame True {
              n545 = global read "全局 小时数据发送次数.vi" "小时数据发送次数"() -> (w846:i32)
              n546 = Increment(x=w846) -> (x+1=w845:i32)
              n547 = global write "全局 小时数据发送次数.vi" "小时数据发送次数"(w845) -> ()
            }
          }
        }
        frame "返回执行结果" {
        }
      }
    }
    frame "提取集成干预" {
      # "提取平行样数据"
      n548 = global read "全局1.vi" "枚举"() -> (w852:enum16{"返回请求应答", "上传数据", "返回执行结果"})
      n549 = case shown="\"上传数据\"" w852 {
        tunnel: ["QnRtn=1" w869 "ExeRtn=1"] -> w851
        tunnel: w850 -> [_ w864 _]
        tunnel: w849 -> [_ w861 _]
        frame "返回请求应答", Default {
          n550 = global read "全局 数据数组大小.vi" "数据数组大小"() -> (w853:i32)
          n551 = Equal To 0?(x=w853) -> (x = 0?=w854:bool)
          n552 = case shown="真" w854 {
            frame False {
            }
            frame True {
              n553 = global read "全局 小时数据发送次数.vi" "小时数据发送次数"() -> (w857:i32)
              n554 = Increment(x=w857) -> (x+1=w856:i32)
              n555 = global write "全局 小时数据发送次数.vi" "小时数据发送次数"(w856) -> ()
            }
          }
        }
        frame "上传数据" {
          # "CODMn"
          n556 = global read "全局 小时数据发送次数.vi" "小时数据发送次数"() -> (w865:i32)
          n557 = call "数据发送组合-20200825 (子VI).vi"("枚举"=T4."集成干预测试", "插值后的数组元素"=w861) -> ("字符串"=w862:string)  [unwired: 9 in]
          n558 = Index Array(array=w864, index (row)=w865) -> (element=w867:string[])  [unwired: 1 in]
          n559 = global read "断电保存全局.vi" "应用环境"() -> (w860:T8)
          n560 = Index Array(array=w867, index=0 ("索引")) -> (element=w859:string)
          n561 = case shown="\"GB212\", 默认" w860 {
            tunnel: [w873 w874] -> w858
            tunnel: w859 -> [w872 w875]
            frame "STD" {
              n562 = call "规范时间戳.vi"("字符串"=w872) -> ("result string"=w873:string)  [unwired: 10 in]
            }
            frame "GB212", Default {
              n563 = call "规范分钟数据时间戳.vi"("字符串"=w875) -> ("result string"=w874:string)  [unwired: 10 in]
            }
          }
          n564 = Empty String/Path?(string/path=w859) -> (empty?=w868:bool)
          n565 = Format Into String(format string="DataTime=%s;%s" ("格式字符串"), w858, w862) -> (resulting string=w870:string)  [unwired: 2 in, 1 out]
          n566 = case shown="真" w868 {
            tunnel: [w878 ""] -> w869
            tunnel: w870 -> [w878 _]
            frame False {
              n567 = global read "全局 小时数据发送次数.vi" "小时数据发送次数"() -> (w877:i32)
              n568 = Increment(x=w877) -> (x+1=w876:i32)
              n569 = global write "全局 小时数据发送次数.vi" "小时数据发送次数"(w876) -> ()
            }
            frame True {
              n570 = global read "全局 小时数据发送次数.vi" "小时数据发送次数"() -> (w880:i32)
              n571 = Increment(x=w880) -> (x+1=w879:i32)
              n572 = global write "全局 小时数据发送次数.vi" "小时数据发送次数"(w879) -> ()
            }
          }
        }
        frame "返回执行结果" {
        }
      }
    }
    frame "操作日志" {
      n573 = global read "全局 小时数据发送次数.vi" "小时数据发送次数"() -> (w885:i32)
      n574 = Index Array(array=w887, index (row)=w885) -> (element=w884:string[])  [unwired: 1 in]
      n575 = global read "全局1.vi" "枚举"() -> (w886:enum16{"返回请求应答", "上传数据", "返回执行结果"})
      n576 = case shown="\"上传数据\"" w886 {
        tunnel: ["QnRtn=1" w905 "ExeRtn=1"] -> w888
        tunnel: w884 -> [_ w907 _]
        tunnel: w883 -> [_ w895 _]
        frame "返回请求应答", Default {
          n577 = global read "全局 数据数组大小.vi" "数据数组大小"() -> (w891:i32)
          n578 = Equal To 0?(x=w891) -> (x = 0?=w890:bool)
          n579 = case shown="真" w890 {
            frame False {
            }
            frame True {
              n580 = global read "全局 小时数据发送次数.vi" "小时数据发送次数"() -> (w893:i32)
              n581 = Increment(x=w893) -> (x+1=w892:i32)
              n582 = global write "全局 小时数据发送次数.vi" "小时数据发送次数"(w892) -> ()
            }
          }
        }
        frame "上传数据" {
          n583 = Index Array(array=w907, index #1=0 ("索引"), index #2=2 ("索引")) -> (element #1=w900:string)  [unwired: 1 out]
          n584 = call "规范时间戳.vi"("字符串"=w900) -> ("result string"=w898:string)  [unwired: 10 in]
          n585 = call "数据发送组合-20200825 (子VI).vi"("枚举"=T5."操作日志", "插值后的数组元素"=w895) -> ("字符串"=w894:string)  [unwired: 9 in]
          n586 = Format Into String(format string="DataTime=%s;", w898) -> (resulting string=w897:string)  [unwired: 2 in, 1 out]
          n587 = Concatenate Strings(w897, w894) -> (w902:string)
          n588 = Empty String/Path?(string/path=w902) -> (empty?=w906:bool)
          n589 = String Length(string=w902) -> (length=w904:i32)
          n590 = Decrement(x=w904) -> (x-1=w903:i32)
          n591 = String Subset(string=w902, length (rest)=w903) -> (substring=w901:string)  [unwired: 1 in]
          n592 = case shown="假" w906 {
            tunnel: [w912 ""] -> w905
            tunnel: w901 -> [w912 _]
            frame False {
              n593 = global read "全局 小时数据发送次数.vi" "小时数据发送次数"() -> (w911:i32)
              n594 = Increment(x=w911) -> (x+1=w910:i32)
              n595 = global write "全局 小时数据发送次数.vi" "小时数据发送次数"(w910) -> ()
            }
            frame True {
              n596 = global read "全局 小时数据发送次数.vi" "小时数据发送次数"() -> (w914:i32)
              n597 = Increment(x=w914) -> (x+1=w913:i32)
              n598 = global write "全局 小时数据发送次数.vi" "小时数据发送次数"(w913) -> ()
            }
          }
        }
        frame "返回执行结果" {
        }
      }
    }
    frame "3092日志信息" {
      n599 = global read "全局 小时数据发送次数.vi" "小时数据发送次数"() -> (w919:i32)
      n600 = global read "全局 所有参数.vi" "CODMn"() -> (w917:string[][])
      n601 = Index Array(array=w917, index (row)=w919) -> (element=w918:string[])  [unwired: 1 in]
      n602 = global read "全局1.vi" "枚举"() -> (w920:enum16{"返回请求应答", "上传数据", "返回执行结果"})
      n603 = case shown="\"上传数据\"" w920 {
        tunnel: ["QnRtn=1" w939 "ExeRtn=1"] -> w921
        tunnel: w918 -> [_ w941 _]
        frame "返回请求应答", Default {
          n604 = global read "全局 数据数组大小.vi" "数据数组大小"() -> (w924:i32)
          n605 = Equal To 0?(x=w924) -> (x = 0?=w923:bool)
          n606 = case shown="真" w923 {
            frame False {
            }
            frame True {
              n607 = global read "全局 小时数据发送次数.vi" "小时数据发送次数"() -> (w926:i32)
              n608 = Increment(x=w926) -> (x+1=w925:i32)
              n609 = global write "全局 小时数据发送次数.vi" "小时数据发送次数"(w925) -> ()
            }
          }
        }
        frame "上传数据" {
          n610 = Index Array(array=w941, index #1=0 ("索引")) -> (element #1=w934:string, element #2=w927:string, element #3=w929:string)  [unwired: 2 in]
          n611 = Empty String/Path?(string/path=w927) -> (empty?=w940:bool)
          n612 = call "规范时间戳.vi"("字符串"=w934) -> ("result string"=w931:string)  [unwired: 10 in]
          n613 = Format Into String(format string="DataTime=%s;", w931) -> (resulting string=w932:string)  [unwired: 2 in, 1 out]
          n614 = Format Into String(format string="parameter=//%s//,content==//%s//;" ("格式字符串"), w927, w929) -> (resulting string=w928:string)  [unwired: 2 in, 1 out]
          n615 = Concatenate Strings(w932, w928) -> (w936:string)
          n616 = String Length(string=w936) -> (length=w938:i32)
          n617 = Decrement(x=w938) -> (x-1=w937:i32)
          n618 = String Subset(string=w936, length (rest)=w937) -> (substring=w935:string)  [unwired: 1 in]
          n619 = case shown="假" w940 {
            tunnel: [w945 ""] -> w939
            tunnel: w935 -> [w945 _]
            frame False {
              n620 = global read "全局 小时数据发送次数.vi" "小时数据发送次数"() -> (w944:i32)
              n621 = Increment(x=w944) -> (x+1=w943:i32)
              n622 = global write "全局 小时数据发送次数.vi" "小时数据发送次数"(w943) -> ()
            }
            frame True {
              n623 = global read "全局 小时数据发送次数.vi" "小时数据发送次数"() -> (w947:i32)
              n624 = Increment(x=w947) -> (x+1=w946:i32)
              n625 = global write "全局 小时数据发送次数.vi" "小时数据发送次数"(w946) -> ()
            }
          }
        }
        frame "返回执行结果" {
        }
      }
    }
    frame "3093报警信息" {
      n626 = global read "全局 小时数据发送次数.vi" "小时数据发送次数"() -> (w952:i32)
      n627 = global read "全局 所有参数.vi" "CODMn"() -> (w950:string[][])
      n628 = Index Array(array=w950, index (row)=w952) -> (element=w951:string[])  [unwired: 1 in]
      n629 = global read "全局1.vi" "枚举"() -> (w953:enum16{"返回请求应答", "上传数据", "返回执行结果"})
      n630 = case shown="\"上传数据\"" w953 {
        tunnel: ["QnRtn=1" w975 "ExeRtn=1"] -> w954
        tunnel: w951 -> [_ w977 _]
        frame "返回请求应答", Default {
          n631 = global read "全局 数据数组大小.vi" "数据数组大小"() -> (w957:i32)
          n632 = Equal To 0?(x=w957) -> (x = 0?=w956:bool)
          n633 = case shown="真" w956 {
            frame False {
            }
            frame True {
              n634 = global read "全局 小时数据发送次数.vi" "小时数据发送次数"() -> (w959:i32)
              n635 = Increment(x=w959) -> (x+1=w958:i32)
              n636 = global write "全局 小时数据发送次数.vi" "小时数据发送次数"(w958) -> ()
            }
          }
        }
        frame "上传数据" {
          n637 = Index Array(array=w977, index #1=0 ("索引")) -> (element #1=w970:string, element #2=w964:string, element #3=w963:string, element #5=w962:string, element #6=w961:string)  [unwired: 5 in, 1 out]
          n638 = case shown="\"产生\"" w961 {
            tunnel: ["0" "1"] -> w960
            frame "消除", Default {
            }
            frame "产生" {
            }
          }
          n639 = Empty String/Path?(string/path=w964) -> (empty?=w976:bool)
          n640 = call "规范时间戳.vi"("字符串"=w970) -> ("result string"=w967:string)  [unwired: 10 in]
          n641 = Format Into String(format string="DataTime=%s;", w967) -> (resulting string=w968:string)  [unwired: 2 in, 1 out]
          n642 = Format Into String(format string="parameter=//%s//,code=//%s//,content=//%s//,state=%s;" ("格式字符串"), w964, w962, w963, w960) -> (resulting string=w965:string)  [unwired: 2 in, 1 out]
          n643 = Concatenate Strings(w968, w965) -> (w972:string)
          n644 = String Length(string=w972) -> (length=w974:i32)
          n645 = Decrement(x=w974) -> (x-1=w973:i32)
          n646 = String Subset(string=w972, length (rest)=w973) -> (substring=w971:string)  [unwired: 1 in]
          n647 = case shown="假" w976 {
            tunnel: [w983 ""] -> w975
            tunnel: w971 -> [w983 _]
            frame False {
              n648 = global read "全局 小时数据发送次数.vi" "小时数据发送次数"() -> (w982:i32)
              n649 = Increment(x=w982) -> (x+1=w981:i32)
              n650 = global write "全局 小时数据发送次数.vi" "小时数据发送次数"(w981) -> ()
            }
            frame True {
              n651 = global read "全局 小时数据发送次数.vi" "小时数据发送次数"() -> (w985:i32)
              n652 = Increment(x=w985) -> (x+1=w984:i32)
              n653 = global write "全局 小时数据发送次数.vi" "小时数据发送次数"(w984) -> ()
            }
          }
        }
        frame "返回执行结果" {
        }
      }
    }
    frame "仪器参数" {
      n654 = case shown="\"氨氮\"" w991 {
        selector: w991 -> [w995 _ _ _ _ _ _ _ _ _ _ _ _ _ _ _ _ _ _ _ _ _ _ _ _ _ _ _ _ _ _ _]
        tunnel: [w995 w998 w1002 w1006 w1010 w1014 w1018 w1022 w1026 w1030 w1034 w1038 w1042 w1046 w1050 w1054 w1058 w1062 w1066 w1070 w1074 w1078 w1082 w1086 w1090 w1094 w1098 w1102 w1106 w1110 w1114 w1118] -> w990
        tunnel: [1.0 ("风向") w996 w1000 w1004 w1008 w1012 w1016 w1020 w1024 w1028 w1032 w1036 w1040 w1044 w1048 w1052 w1056 w1060 w1064 w1068 w1072 w1076 w1080 w1084 w1088 w1092 w1096 w1100 w1104 w1108 w1112 w1116] -> _
        frame "假", Default {
        }
        frame "CODMn" {
          n655 = global read "断电保存全局.vi" "参数系数簇"() -> (w997:T9)
          n656 = global read "断电保存全局.vi" "因子编码簇"() -> (w999:T10)
          n657 = Unbundle By Name(w997) -> ("CODMn"=w996:dbl)
          n658 = Unbundle By Name(w999) -> ("CODMn"=w998:string)
        }
        frame "CODCr" {
          n659 = global read "断电保存全局.vi" "参数系数簇"() -> (w1001:T9)
          n660 = global read "断电保存全局.vi" "因子编码簇"() -> (w1003:T10)
          n661 = Unbundle By Name(w1001) -> ("CODCr"=w1000:dbl)
          n662 = Unbundle By Name(w1003) -> ("CODCr"=w1002:string)
        }
        frame "DO" {
          n663 = global read "断电保存全局.vi" "参数系数簇"() -> (w1005:T9)
          n664 = global read "断电保存全局.vi" "因子编码簇"() -> (w1007:T10)
          n665 = Unbundle By Name(w1005) -> ("DO"=w1004:dbl)
          n666 = Unbundle By Name(w1007) -> ("DO"=w1006:string)
        }
        frame "铜" {
          n667 = global read "断电保存全局.vi" "参数系数簇"() -> (w1009:T9)
          n668 = global read "断电保存全局.vi" "因子编码簇"() -> (w1011:T10)
          n669 = Unbundle By Name(w1009) -> ("铜"=w1008:dbl)
          n670 = Unbundle By Name(w1011) -> ("铜"=w1010:string)
        }
        frame "PH" {
          n671 = global read "断电保存全局.vi" "参数系数簇"() -> (w1013:T9)
          n672 = global read "断电保存全局.vi" "因子编码簇"() -> (w1015:T10)
          n673 = Unbundle By Name(w1013) -> ("PH"=w1012:dbl)
          n674 = Unbundle By Name(w1015) -> ("PH"=w1014:string)
        }
        frame "氨氮" {
          n675 = global read "断电保存全局.vi" "参数系数簇"() -> (w1017:T9)
          n676 = global read "断电保存全局.vi" "因子编码簇"() -> (w1019:T10)
          n677 = Unbundle By Name(w1017) -> ("氨氮"=w1016:dbl)
          n678 = Unbundle By Name(w1019) -> ("氨氮"=w1018:string)
        }
        frame "比电导率" {
          n679 = global read "断电保存全局.vi" "参数系数簇"() -> (w1021:T9)
          n680 = global read "断电保存全局.vi" "因子编码簇"() -> (w1023:T10)
          n681 = Unbundle By Name(w1021) -> ("比电导率"=w1020:dbl)
          n682 = Unbundle By Name(w1023) -> ("比电导率"=w1022:string)
        }
        frame "水温" {
          n683 = global read "断电保存全局.vi" "参数系数簇"() -> (w1025:T9)
          n684 = global read "断电保存全局.vi" "因子编码簇"() -> (w1027:T10)
          n685 = Unbundle By Name(w1025) -> ("水温"=w1024:dbl)
          n686 = Unbundle By Name(w1027) -> ("水温"=w1026:string)
        }
        frame "COD" {
          n687 = global read "断电保存全局.vi" "参数系数簇"() -> (w1029:T9)
          n688 = global read "断电保存全局.vi" "因子编码簇"() -> (w1031:T10)
          n689 = Unbundle By Name(w1029) -> ("COD"=w1028:dbl)
          n690 = Unbundle By Name(w1031) -> ("COD"=w1030:string)
        }
        frame "浊度" {
          n691 = global read "断电保存全局.vi" "参数系数簇"() -> (w1033:T9)
          n692 = global read "断电保存全局.vi" "因子编码簇"() -> (w1035:T10)
          n693 = Unbundle By Name(w1033) -> ("浊度"=w1032:dbl)
          n694 = Unbundle By Name(w1035) -> ("浊度"=w1034:string)
        }
        frame "总氮" {
          n695 = global read "断电保存全局.vi" "参数系数簇"() -> (w1037:T9)
          n696 = global read "断电保存全局.vi" "因子编码簇"() -> (w1039:T10)
          n697 = Unbundle By Name(w1037) -> ("总氮"=w1036:dbl)
          n698 = Unbundle By Name(w1039) -> ("总氮"=w1038:string)
        }
        frame "总磷" {
          n699 = global read "断电保存全局.vi" "参数系数簇"() -> (w1041:T9)
          n700 = global read "断电保存全局.vi" "因子编码簇"() -> (w1043:T10)
          n701 = Unbundle By Name(w1041) -> ("总磷"=w1040:dbl)
          n702 = Unbundle By Name(w1043) -> ("总磷"=w1042:string)
        }
        frame "叶绿素a" {
          n703 = global read "断电保存全局.vi" "参数系数簇"() -> (w1045:T9)
          n704 = global read "断电保存全局.vi" "因子编码簇"() -> (w1047:T10)
          n705 = Unbundle By Name(w1045) -> ("叶绿素a"=w1044:dbl)
          n706 = Unbundle By Name(w1047) -> ("叶绿素a"=w1046:string)
        }
        frame "藻密度" {
          n707 = global read "断电保存全局.vi" "参数系数簇"() -> (w1049:T9)
          n708 = global read "断电保存全局.vi" "因子编码簇"() -> (w1051:T10)
          n709 = Unbundle By Name(w1049) -> ("藻密度"=w1048:dbl)
          n710 = Unbundle By Name(w1051) -> ("藻密度"=w1050:string)
        }
        frame "水位" {
          n711 = global read "断电保存全局.vi" "参数系数簇"() -> (w1053:T9)
          n712 = global read "断电保存全局.vi" "因子编码簇"() -> (w1055:T10)
          n713 = Unbundle By Name(w1053) -> ("水位"=w1052:dbl)
          n714 = Unbundle By Name(w1055) -> ("水位"=w1054:string)
        }
        frame "流速" {
          n715 = global read "断电保存全局.vi" "参数系数簇"() -> (w1057:T9)
          n716 = global read "断电保存全局.vi" "因子编码簇"() -> (w1059:T10)
          n717 = Unbundle By Name(w1057) -> ("流速"=w1056:dbl)
          n718 = Unbundle By Name(w1059) -> ("流速"=w1058:string)
        }
        frame "瞬时流量" {
          n719 = global read "断电保存全局.vi" "参数系数簇"() -> (w1061:T9)
          n720 = global read "断电保存全局.vi" "因子编码簇"() -> (w1063:T10)
          n721 = Unbundle By Name(w1061) -> ("瞬时流量"=w1060:dbl)
          n722 = Unbundle By Name(w1063) -> ("瞬时流量"=w1062:string)
        }
        frame "累积流量" {
          n723 = global read "断电保存全局.vi" "参数系数簇"() -> (w1065:T9)
          n724 = global read "断电保存全局.vi" "因子编码簇"() -> (w1067:T10)
          n725 = Unbundle By Name(w1065) -> ("累积流量"=w1064:dbl)
          n726 = Unbundle By Name(w1067) -> ("累积流量"=w1066:string)
        }
        frame "亚硝酸盐" {
          n727 = global read "断电保存全局.vi" "参数系数簇"() -> (w1069:T9)
          n728 = global read "断电保存全局.vi" "因子编码簇"() -> (w1071:T10)
          n729 = Unbundle By Name(w1069) -> ("亚硝酸盐"=w1068:dbl)
          n730 = Unbundle By Name(w1071) -> ("亚硝酸盐"=w1070:string)
        }
        frame "硫化物" {
          n731 = global read "断电保存全局.vi" "参数系数簇"() -> (w1073:T9)
          n732 = global read "断电保存全局.vi" "因子编码簇"() -> (w1075:T10)
          n733 = Unbundle By Name(w1073) -> ("硫化物"=w1072:dbl)
          n734 = Unbundle By Name(w1075) -> ("硫化物"=w1074:string)
        }
        frame "ORP" {
          n735 = global read "断电保存全局.vi" "参数系数簇"() -> (w1077:T9)
          n736 = global read "断电保存全局.vi" "因子编码簇"() -> (w1079:T10)
          n737 = Unbundle By Name(w1077) -> ("ORP"=w1076:dbl)
          n738 = Unbundle By Name(w1079) -> ("ORP"=w1078:string)
        }
        frame "铅" {
          n739 = global read "断电保存全局.vi" "参数系数簇"() -> (w1081:T9)
          n740 = global read "断电保存全局.vi" "因子编码簇"() -> (w1083:T10)
          n741 = Unbundle By Name(w1081) -> ("铅"=w1080:dbl)
          n742 = Unbundle By Name(w1083) -> ("铅"=w1082:string)
        }
        frame "镉" {
          n743 = global read "断电保存全局.vi" "参数系数簇"() -> (w1085:T9)
          n744 = global read "断电保存全局.vi" "因子编码簇"() -> (w1087:T10)
          n745 = Unbundle By Name(w1085) -> ("镉"=w1084:dbl)
          n746 = Unbundle By Name(w1087) -> ("镉"=w1086:string)
        }
        frame "锌" {
          n747 = global read "断电保存全局.vi" "参数系数簇"() -> (w1089:T9)
          n748 = global read "断电保存全局.vi" "因子编码簇"() -> (w1091:T10)
          n749 = Unbundle By Name(w1089) -> ("锌"=w1088:dbl)
          n750 = Unbundle By Name(w1091) -> ("锌"=w1090:string)
        }
        frame "镍" {
          n751 = global read "断电保存全局.vi" "参数系数簇"() -> (w1093:T9)
          n752 = global read "断电保存全局.vi" "因子编码簇"() -> (w1095:T10)
          n753 = Unbundle By Name(w1093) -> ("镍"=w1092:dbl)
          n754 = Unbundle By Name(w1095) -> ("镍"=w1094:string)
        }
        frame "锰" {
          n755 = global read "断电保存全局.vi" "参数系数簇"() -> (w1097:T9)
          n756 = global read "断电保存全局.vi" "因子编码簇"() -> (w1099:T10)
          n757 = Unbundle By Name(w1097) -> ("锰"=w1096:dbl)
          n758 = Unbundle By Name(w1099) -> ("锰"=w1098:string)
        }
        frame "汞" {
          n759 = global read "断电保存全局.vi" "参数系数簇"() -> (w1101:T9)
          n760 = global read "断电保存全局.vi" "因子编码簇"() -> (w1103:T10)
          n761 = Unbundle By Name(w1101) -> ("汞"=w1100:dbl)
          n762 = Unbundle By Name(w1103) -> ("汞"=w1102:string)
        }
        frame "气温" {
          n763 = global read "断电保存全局.vi" "参数系数簇"() -> (w1105:T9)
          n764 = global read "断电保存全局.vi" "因子编码簇"() -> (w1107:T10)
          n765 = Unbundle By Name(w1105) -> ("气温"=w1104:dbl)
          n766 = Unbundle By Name(w1107) -> ("气温"=w1106:string)
        }
        frame "气压" {
          n767 = global read "断电保存全局.vi" "参数系数簇"() -> (w1109:T9)
          n768 = global read "断电保存全局.vi" "因子编码簇"() -> (w1111:T10)
          n769 = Unbundle By Name(w1109) -> ("气压"=w1108:dbl)
          n770 = Unbundle By Name(w1111) -> ("气压"=w1110:string)
        }
        frame "风速" {
          n771 = global read "断电保存全局.vi" "参数系数簇"() -> (w1113:T9)
          n772 = global read "断电保存全局.vi" "因子编码簇"() -> (w1115:T10)
          n773 = Unbundle By Name(w1113) -> ("风速"=w1112:dbl)
          n774 = Unbundle By Name(w1115) -> ("风速"=w1114:string)
        }
        frame "风向" {
          n775 = global read "断电保存全局.vi" "参数系数簇"() -> (w1117:T9)
          n776 = global read "断电保存全局.vi" "因子编码簇"() -> (w1119:T10)
          n777 = Unbundle By Name(w1117) -> ("风向"=w1116:dbl)
          n778 = Unbundle By Name(w1119) -> ("风向"=w1118:string)
        }
      }
      n779 = global read "全局1.vi" "枚举"() -> (w992:enum16{"返回请求应答", "上传数据", "返回执行结果"})
      n780 = case shown="\"上传数据\"" w992 {
        tunnel: ["QnRtn=1" w1137 "ExeRtn=1"] -> w993
        tunnel: w989 -> [_ w1129 _]
        tunnel: w990 -> [_ w1128 _]
        tunnel: w988 -> [_ w1126 _]
        frame "返回请求应答", Default {
          n781 = global read "全局 数据数组大小.vi" "数据数组大小"() -> (w1122:i32)
          n782 = Equal To 0?(x=w1122) -> (x = 0?=w1121:bool)
          n783 = case shown="真" w1121 {
            frame False {
            }
            frame True {
              n784 = global read "全局 小时数据发送次数.vi" "小时数据发送次数"() -> (w1124:i32)
              n785 = Increment(x=w1124) -> (x+1=w1123:i32)
              n786 = global write "全局 小时数据发送次数.vi" "小时数据发送次数"(w1123) -> ()
            }
          }
        }
        frame "上传数据" {
          n787 = Index Array(array=w1129) -> (element=w1130:string)  [unwired: 1 in]
          n788 = case shown="\"原始时间\"" w1126 {
            tunnel: [w1140 w1142] -> w1131
            tunnel: w1130 -> [w1139 w1141]
            frame "精确到小时", Default {
              n789 = call "规范小时时间戳.vi"("字符串"=w1139) -> ("result string"=w1140:string)  [unwired: 10 in]
            }
            frame "原始时间" {
              n790 = call "日期字符串格式至时间格式转换(子VI).vi"("data[0]"=w1141) -> ("time stamp"=w1144:timestamp)  [unwired: 10 in]
              n791 = Seconds To Date/Time(time stamp (now)=w1144) -> (date time rec=w1143:T11)  [unwired: 1 in]
              n792 = Date/Time To Seconds(2:w1143) -> (0:w1145:timestamp)  [unwired: 1 in]
              n793 = Format Date/Time String(time format string (%c)="%Y%m%d%H%M%S" ("时间格式字符串(%c)"), seconds (now)=w1145) -> (date/time string=w1142:string)  [unwired: 1 in]
            }
          }
          n794 = call "关键参数组合 (子VI).vi"("table"="仪器参数", "因子编码"=w1128, "data"=w1129) -> ("字符串"=w1125:string)  [unwired: 8 in]
          n795 = Empty String/Path?(string/path=w1125) -> (empty?=w1138:bool)
          n796 = Format Into String(format string="DataTime=%s;%s" ("格式字符串"), w1131, w1125) -> (resulting string=w1133:string)  [unwired: 2 in, 1 out]
          n797 = String Length(string=w1133) -> (length=w1134:i32)
          n798 = Decrement(x=w1134) -> (x-1=w1135:i32)
          n799 = String Subset(string=w1133, length (rest)=w1135) -> (substring=w1132:string)  [unwired: 1 in]
          n800 = case shown="假" w1138 {
            tunnel: [w1147 ""] -> w1137
            tunnel: w1132 -> [w1147 _]
            frame False {
            }
            frame True {
            }
          }
        }
        frame "返回执行结果" {
        }
      }
    }
    frame "采配水仪器参数" {
      n801 = global read "全局1.vi" "枚举"() -> (w1153:enum16{"返回请求应答", "上传数据", "返回执行结果"})
      n802 = case shown="\"上传数据\"" w1153 {
        tunnel: ["QnRtn=1" w1178 "ExeRtn=1"] -> w1154
        tunnel: w1152 -> [_ w1166 _]
        tunnel: "w00000" -> [_ w1167 _]
        tunnel: w1151 -> [_ w1170 _]
        frame "返回请求应答", Default {
          n803 = global read "全局 数据数组大小.vi" "数据数组大小"() -> (w1157:i32)
          n804 = Equal To 0?(x=w1157) -> (x = 0?=w1156:bool)
          n805 = case shown="真" w1156 {
            frame False {
            }
            frame True {
              n806 = global read "全局 小时数据发送次数.vi" "小时数据发送次数"() -> (w1159:i32)
              n807 = Increment(x=w1159) -> (x+1=w1158:i32)
              n808 = global write "全局 小时数据发送次数.vi" "小时数据发送次数"(w1158) -> ()
            }
          }
        }
        frame "上传数据" {
          n809 = Index Array(array=w1166) -> (element=w1171:string)  [unwired: 1 in]
          n810 = case shown="\"原始时间\"" w1170 {
            tunnel: [w1181 w1183] -> w1172
            tunnel: w1171 -> [w1180 w1182]
            frame "精确到小时", Default {
              n811 = call "规范小时时间戳.vi"("字符串"=w1180) -> ("result string"=w1181:string)  [unwired: 10 in]
            }
            frame "原始时间" {
              n812 = call "日期字符串格式至时间格式转换(子VI).vi"("data[0]"=w1182) -> ("time stamp"=w1185:timestamp)  [unwired: 10 in]
              n813 = Seconds To Date/Time(time stamp (now)=w1185) -> (date time rec=w1184:T11)  [unwired: 1 in]
              n814 = Date/Time To Seconds(2:w1184) -> (0:w1186:timestamp)  [unwired: 1 in]
              n815 = Format Date/Time String(time format string (%c)="%Y%m%d%H%M%S" ("时间格式字符串(%c)"), seconds (now)=w1186) -> (date/time string=w1183:string)  [unwired: 1 in]
            }
          }
          n816 = Index Array(array=w1166, index #1=2 ("索引"), index #2=3 ("索引"), index #3=4 ("索引")) -> (element #1=w1162:string, element #2=w1161:string, element #3=w1160:string)
          n817 = Format Into String(format string="PolId=%s,i13111-Info=%s,i13112-Info=%s,i13113-Info=%s;", w1167, w1162, w1161, w1160) -> (resulting string=w1168:string)  [unwired: 2 in, 1 out]
          n818 = Empty String/Path?(string/path=w1168) -> (empty?=w1179:bool)
          n819 = Format Into String(format string="DataTime=%s;%s" ("格式字符串"), w1172, w1168) -> (resulting string=w1174:string)  [unwired: 2 in, 1 out]
          n820 = String Length(string=w1174) -> (length=w1175:i32)
          n821 = Decrement(x=w1175) -> (x-1=w1176:i32)
          n822 = String Subset(string=w1174, length (rest)=w1176) -> (substring=w1173:string)  [unwired: 1 in]
          n823 = case shown="假" w1179 {
            tunnel: [w1188 ""] -> w1178
            tunnel: w1173 -> [w1188 _]
            frame False {
            }
            frame True {
            }
          }
        }
        frame "返回执行结果" {
        }
      }
    }
    frame "3091校准信息" {
      n824 = case shown="\"CODMn\"" w1194 {
        selector: w1194 -> [w1198 _ _ _ _ _ _ _ _ _ _ _ _ _ _ _ _ _ _ _ _ _ _ _ _ _ _ _ _ _ _ _]
        tunnel: [w1198 w1201 w1205 w1209 w1213 w1217 w1221 w1225 w1229 w1233 w1237 w1241 w1245 w1249 w1253 w1257 w1261 w1265 w1269 w1273 w1277 w1281 w1285 w1289 w1293 w1297 w1301 w1305 w1309 w1313 w1317 w1321] -> w1193
        tunnel: [1.0 ("风向") w1199 w1203 w1207 w1211 w1215 w1219 w1223 w1227 w1231 w1235 w1239 w1243 w1247 w1251 w1255 w1259 w1263 w1267 w1271 w1275 w1279 w1283 w1287 w1291 w1295 w1299 w1303 w1307 w1311 w1315 w1319] -> _
        frame "假", Default {
        }
        frame "CODMn" {
          n825 = global read "断电保存全局.vi" "参数系数簇"() -> (w1200:T9)
          n826 = global read "断电保存全局.vi" "因子编码簇"() -> (w1202:T10)
          n827 = Unbundle By Name(w1200) -> ("CODMn"=w1199:dbl)
          n828 = Unbundle By Name(w1202) -> ("CODMn"=w1201:string)
        }
        frame "CODCr" {
          n829 = global read "断电保存全局.vi" "参数系数簇"() -> (w1204:T9)
          n830 = global read "断电保存全局.vi" "因子编码簇"() -> (w1206:T10)
          n831 = Unbundle By Name(w1204) -> ("CODCr"=w1203:dbl)
          n832 = Unbundle By Name(w1206) -> ("CODCr"=w1205:string)
        }
        frame "DO" {
          n833 = global read "断电保存全局.vi" "参数系数簇"() -> (w1208:T9)
          n834 = global read "断电保存全局.vi" "因子编码簇"() -> (w1210:T10)
          n835 = Unbundle By Name(w1208) -> ("DO"=w1207:dbl)
          n836 = Unbundle By Name(w1210) -> ("DO"=w1209:string)
        }
        frame "铜" {
          n837 = global read "断电保存全局.vi" "参数系数簇"() -> (w1212:T9)
          n838 = global read "断电保存全局.vi" "因子编码簇"() -> (w1214:T10)
          n839 = Unbundle By Name(w1212) -> ("铜"=w1211:dbl)
          n840 = Unbundle By Name(w1214) -> ("铜"=w1213:string)
        }
        frame "PH" {
          n841 = global read "断电保存全局.vi" "参数系数簇"() -> (w1216:T9)
          n842 = global read "断电保存全局.vi" "因子编码簇"() -> (w1218:T10)
          n843 = Unbundle By Name(w1216) -> ("PH"=w1215:dbl)
          n844 = Unbundle By Name(w1218) -> ("PH"=w1217:string)
        }
        frame "氨氮" {
          n845 = global read "断电保存全局.vi" "参数系数簇"() -> (w1220:T9)
          n846 = global read "断电保存全局.vi" "因子编码簇"() -> (w1222:T10)
          n847 = Unbundle By Name(w1220) -> ("氨氮"=w1219:dbl)
          n848 = Unbundle By Name(w1222) -> ("氨氮"=w1221:string)
        }
        frame "比电导率" {
          n849 = global read "断电保存全局.vi" "参数系数簇"() -> (w1224:T9)
          n850 = global read "断电保存全局.vi" "因子编码簇"() -> (w1226:T10)
          n851 = Unbundle By Name(w1224) -> ("比电导率"=w1223:dbl)
          n852 = Unbundle By Name(w1226) -> ("比电导率"=w1225:string)
        }
        frame "水温" {
          n853 = global read "断电保存全局.vi" "参数系数簇"() -> (w1228:T9)
          n854 = global read "断电保存全局.vi" "因子编码簇"() -> (w1230:T10)
          n855 = Unbundle By Name(w1228) -> ("水温"=w1227:dbl)
          n856 = Unbundle By Name(w1230) -> ("水温"=w1229:string)
        }
        frame "COD" {
          n857 = global read "断电保存全局.vi" "参数系数簇"() -> (w1232:T9)
          n858 = global read "断电保存全局.vi" "因子编码簇"() -> (w1234:T10)
          n859 = Unbundle By Name(w1232) -> ("COD"=w1231:dbl)
          n860 = Unbundle By Name(w1234) -> ("COD"=w1233:string)
        }
        frame "浊度" {
          n861 = global read "断电保存全局.vi" "参数系数簇"() -> (w1236:T9)
          n862 = global read "断电保存全局.vi" "因子编码簇"() -> (w1238:T10)
          n863 = Unbundle By Name(w1236) -> ("浊度"=w1235:dbl)
          n864 = Unbundle By Name(w1238) -> ("浊度"=w1237:string)
        }
        frame "总氮" {
          n865 = global read "断电保存全局.vi" "参数系数簇"() -> (w1240:T9)
          n866 = global read "断电保存全局.vi" "因子编码簇"() -> (w1242:T10)
          n867 = Unbundle By Name(w1240) -> ("总氮"=w1239:dbl)
          n868 = Unbundle By Name(w1242) -> ("总氮"=w1241:string)
        }
        frame "总磷" {
          n869 = global read "断电保存全局.vi" "参数系数簇"() -> (w1244:T9)
          n870 = global read "断电保存全局.vi" "因子编码簇"() -> (w1246:T10)
          n871 = Unbundle By Name(w1244) -> ("总磷"=w1243:dbl)
          n872 = Unbundle By Name(w1246) -> ("总磷"=w1245:string)
        }
        frame "叶绿素a" {
          n873 = global read "断电保存全局.vi" "参数系数簇"() -> (w1248:T9)
          n874 = global read "断电保存全局.vi" "因子编码簇"() -> (w1250:T10)
          n875 = Unbundle By Name(w1248) -> ("叶绿素a"=w1247:dbl)
          n876 = Unbundle By Name(w1250) -> ("叶绿素a"=w1249:string)
        }
        frame "藻密度" {
          n877 = global read "断电保存全局.vi" "参数系数簇"() -> (w1252:T9)
          n878 = global read "断电保存全局.vi" "因子编码簇"() -> (w1254:T10)
          n879 = Unbundle By Name(w1252) -> ("藻密度"=w1251:dbl)
          n880 = Unbundle By Name(w1254) -> ("藻密度"=w1253:string)
        }
        frame "水位" {
          n881 = global read "断电保存全局.vi" "参数系数簇"() -> (w1256:T9)
          n882 = global read "断电保存全局.vi" "因子编码簇"() -> (w1258:T10)
          n883 = Unbundle By Name(w1256) -> ("水位"=w1255:dbl)
          n884 = Unbundle By Name(w1258) -> ("水位"=w1257:string)
        }
        frame "流速" {
          n885 = global read "断电保存全局.vi" "参数系数簇"() -> (w1260:T9)
          n886 = global read "断电保存全局.vi" "因子编码簇"() -> (w1262:T10)
          n887 = Unbundle By Name(w1260) -> ("流速"=w1259:dbl)
          n888 = Unbundle By Name(w1262) -> ("流速"=w1261:string)
        }
        frame "瞬时流量" {
          n889 = global read "断电保存全局.vi" "参数系数簇"() -> (w1264:T9)
          n890 = global read "断电保存全局.vi" "因子编码簇"() -> (w1266:T10)
          n891 = Unbundle By Name(w1264) -> ("瞬时流量"=w1263:dbl)
          n892 = Unbundle By Name(w1266) -> ("瞬时流量"=w1265:string)
        }
        frame "累积流量" {
          n893 = global read "断电保存全局.vi" "参数系数簇"() -> (w1268:T9)
          n894 = global read "断电保存全局.vi" "因子编码簇"() -> (w1270:T10)
          n895 = Unbundle By Name(w1268) -> ("累积流量"=w1267:dbl)
          n896 = Unbundle By Name(w1270) -> ("累积流量"=w1269:string)
        }
        frame "亚硝酸盐" {
          n897 = global read "断电保存全局.vi" "参数系数簇"() -> (w1272:T9)
          n898 = global read "断电保存全局.vi" "因子编码簇"() -> (w1274:T10)
          n899 = Unbundle By Name(w1272) -> ("亚硝酸盐"=w1271:dbl)
          n900 = Unbundle By Name(w1274) -> ("亚硝酸盐"=w1273:string)
        }
        frame "硫化物" {
          n901 = global read "断电保存全局.vi" "参数系数簇"() -> (w1276:T9)
          n902 = global read "断电保存全局.vi" "因子编码簇"() -> (w1278:T10)
          n903 = Unbundle By Name(w1276) -> ("硫化物"=w1275:dbl)
          n904 = Unbundle By Name(w1278) -> ("硫化物"=w1277:string)
        }
        frame "ORP" {
          n905 = global read "断电保存全局.vi" "参数系数簇"() -> (w1280:T9)
          n906 = global read "断电保存全局.vi" "因子编码簇"() -> (w1282:T10)
          n907 = Unbundle By Name(w1280) -> ("ORP"=w1279:dbl)
          n908 = Unbundle By Name(w1282) -> ("ORP"=w1281:string)
        }
        frame "铅" {
          n909 = global read "断电保存全局.vi" "参数系数簇"() -> (w1284:T9)
          n910 = global read "断电保存全局.vi" "因子编码簇"() -> (w1286:T10)
          n911 = Unbundle By Name(w1284) -> ("铅"=w1283:dbl)
          n912 = Unbundle By Name(w1286) -> ("铅"=w1285:string)
        }
        frame "镉" {
          n913 = global read "断电保存全局.vi" "参数系数簇"() -> (w1288:T9)
          n914 = global read "断电保存全局.vi" "因子编码簇"() -> (w1290:T10)
          n915 = Unbundle By Name(w1288) -> ("镉"=w1287:dbl)
          n916 = Unbundle By Name(w1290) -> ("镉"=w1289:string)
        }
        frame "锌" {
          n917 = global read "断电保存全局.vi" "参数系数簇"() -> (w1292:T9)
          n918 = global read "断电保存全局.vi" "因子编码簇"() -> (w1294:T10)
          n919 = Unbundle By Name(w1292) -> ("锌"=w1291:dbl)
          n920 = Unbundle By Name(w1294) -> ("锌"=w1293:string)
        }
        frame "镍" {
          n921 = global read "断电保存全局.vi" "参数系数簇"() -> (w1296:T9)
          n922 = global read "断电保存全局.vi" "因子编码簇"() -> (w1298:T10)
          n923 = Unbundle By Name(w1296) -> ("镍"=w1295:dbl)
          n924 = Unbundle By Name(w1298) -> ("镍"=w1297:string)
        }
        frame "锰" {
          n925 = global read "断电保存全局.vi" "参数系数簇"() -> (w1300:T9)
          n926 = global read "断电保存全局.vi" "因子编码簇"() -> (w1302:T10)
          n927 = Unbundle By Name(w1300) -> ("锰"=w1299:dbl)
          n928 = Unbundle By Name(w1302) -> ("锰"=w1301:string)
        }
        frame "汞" {
          n929 = global read "断电保存全局.vi" "参数系数簇"() -> (w1304:T9)
          n930 = global read "断电保存全局.vi" "因子编码簇"() -> (w1306:T10)
          n931 = Unbundle By Name(w1304) -> ("汞"=w1303:dbl)
          n932 = Unbundle By Name(w1306) -> ("汞"=w1305:string)
        }
        frame "气温" {
          n933 = global read "断电保存全局.vi" "参数系数簇"() -> (w1308:T9)
          n934 = global read "断电保存全局.vi" "因子编码簇"() -> (w1310:T10)
          n935 = Unbundle By Name(w1308) -> ("气温"=w1307:dbl)
          n936 = Unbundle By Name(w1310) -> ("气温"=w1309:string)
        }
        frame "气压" {
          n937 = global read "断电保存全局.vi" "参数系数簇"() -> (w1312:T9)
          n938 = global read "断电保存全局.vi" "因子编码簇"() -> (w1314:T10)
          n939 = Unbundle By Name(w1312) -> ("气压"=w1311:dbl)
          n940 = Unbundle By Name(w1314) -> ("气压"=w1313:string)
        }
        frame "风速" {
          n941 = global read "断电保存全局.vi" "参数系数簇"() -> (w1316:T9)
          n942 = global read "断电保存全局.vi" "因子编码簇"() -> (w1318:T10)
          n943 = Unbundle By Name(w1316) -> ("风速"=w1315:dbl)
          n944 = Unbundle By Name(w1318) -> ("风速"=w1317:string)
        }
        frame "风向" {
          n945 = global read "断电保存全局.vi" "参数系数簇"() -> (w1320:T9)
          n946 = global read "断电保存全局.vi" "因子编码簇"() -> (w1322:T10)
          n947 = Unbundle By Name(w1320) -> ("风向"=w1319:dbl)
          n948 = Unbundle By Name(w1322) -> ("风向"=w1321:string)
        }
      }
      n949 = global read "全局1.vi" "枚举"() -> (w1195:enum16{"返回请求应答", "上传数据", "返回执行结果"})
      n950 = case shown="\"上传数据\"" w1195 {
        tunnel: ["QnRtn=1" w1339 "ExeRtn=1"] -> w1196
        tunnel: w1192 -> [_ w1329 _]
        tunnel: w1193 -> [_ w1328 _]
        tunnel: w1191 -> [_ w1331 _]
        frame "返回请求应答", Default {
          n951 = global read "全局 数据数组大小.vi" "数据数组大小"() -> (w1325:i32)
          n952 = Equal To 0?(x=w1325) -> (x = 0?=w1324:bool)
          n953 = case shown="真" w1324 {
            frame False {
            }
            frame True {
              n954 = global read "全局 小时数据发送次数.vi" "小时数据发送次数"() -> (w1327:i32)
              n955 = Increment(x=w1327) -> (x+1=w1326:i32)
              n956 = global write "全局 小时数据发送次数.vi" "小时数据发送次数"(w1326) -> ()
            }
          }
        }
        frame "上传数据" {
          n957 = call "校准信息组合 (子VI).vi"("因子编码"=w1328, "data"=w1329) -> ("字符串"=w1330:string)  [unwired: 9 in]
          n958 = Index Array(array=w1329) -> (element=w1332:string)  [unwired: 1 in]
          n959 = case shown="\"原始时间\"" w1331 {
            tunnel: [w1342 w1344] -> w1333
            tunnel: w1332 -> [w1341 w1343]
            frame "精确到小时", Default {
              n960 = call "规范小时时间戳.vi"("字符串"=w1341) -> ("result string"=w1342:string)  [unwired: 10 in]
            }
            frame "原始时间" {
              n961 = call "日期字符串格式至时间格式转换(子VI).vi"("data[0]"=w1343) -> ("time stamp"=w1346:timestamp)  [unwired: 10 in]
              n962 = Seconds To Date/Time(time stamp (now)=w1346) -> (date time rec=w1345:T11)  [unwired: 1 in]
              n963 = Date/Time To Seconds(2:w1345) -> (0:w1347:timestamp)  [unwired: 1 in]
              n964 = Format Date/Time String(time format string (%c)="%Y%m%d%H%M%S" ("时间格式字符串(%c)"), seconds (now)=w1347) -> (date/time string=w1344:string)  [unwired: 1 in]
            }
          }
          n965 = Empty String/Path?(string/path=w1330) -> (empty?=w1340:bool)
          n966 = Format Into String(format string="DataTime=%s;%s" ("格式字符串"), w1333, w1330) -> (resulting string=w1335:string)  [unwired: 2 in, 1 out]
          n967 = String Length(string=w1335) -> (length=w1336:i32)
          n968 = Decrement(x=w1336) -> (x-1=w1337:i32)
          n969 = String Subset(string=w1335, length (rest)=w1337) -> (substring=w1334:string)  [unwired: 1 in]
          n970 = case shown="假" w1340 {
            tunnel: [w1349 ""] -> w1339
            tunnel: w1334 -> [w1349 _]
            frame False {
            }
            frame True {
            }
          }
        }
        frame "返回执行结果" {
        }
      }
    }
    frame "3090仪器参数" {
      n971 = global read "全局 小时数据发送次数.vi" "小时数据发送次数"() -> (w1354:i32)
      n972 = Index Array(array=w1356, index (row)=w1354) -> (element=w1353:string[])  [unwired: 1 in]
      n973 = global read "全局1.vi" "枚举"() -> (w1355:enum16{"返回请求应答", "上传数据", "返回执行结果"})
      n974 = case shown="\"上传数据\"" w1355 {
        tunnel: ["QnRtn=1" w1374 "ExeRtn=1"] -> w1357
        tunnel: w1353 -> [_ w1371 _]
        tunnel: w1352 -> [_ w1364 _]
        frame "返回请求应答", Default {
          n975 = global read "全局 数据数组大小.vi" "数据数组大小"() -> (w1360:i32)
          n976 = Equal To 0?(x=w1360) -> (x = 0?=w1359:bool)
          n977 = case shown="真" w1359 {
            frame False {
            }
            frame True {
              n978 = global read "全局 小时数据发送次数.vi" "小时数据发送次数"() -> (w1362:i32)
              n979 = Increment(x=w1362) -> (x+1=w1361:i32)
              n980 = global write "全局 小时数据发送次数.vi" "小时数据发送次数"(w1361) -> ()
            }
          }
        }
        frame "上传数据" {
          n981 = Index Array(array=w1371) -> (element=w1370:string)  [unwired: 1 in]
          n982 = call "数据发送组合-20200825 (子VI).vi"("枚举"=T6."3090仪器参数", "插值后的数组元素"=w1364) -> ("字符串"=w1363:string)  [unwired: 9 in]
          n983 = call "规范时间戳.vi"("字符串"=w1370) -> ("result string"=w1372:string)  [unwired: 10 in]
          n984 = Format Into String(format string="DataTime=%s;%s" ("格式字符串"), w1372, w1363) -> (resulting string=w1367:string)  [unwired: 2 in, 1 out]
          n985 = String Length(string=w1367) -> (length=w1368:i32)
          n986 = Decrement(x=w1368) -> (x-1=w1369:i32)
          n987 = String Subset(string=w1367, length (rest)=w1369) -> (substring=w1366:string)  [unwired: 1 in]
          n988 = Empty String/Path?(string/path=w1366) -> (empty?=w1375:bool)
          n989 = case shown="假" w1375 {
            tunnel: [w1378 ""] -> w1374
            tunnel: w1366 -> [w1378 _]
            frame False {
              n990 = global read "全局 小时数据发送次数.vi" "小时数据发送次数"() -> (w1377:i32)
              n991 = Increment(x=w1377) -> (x+1=w1376:i32)
              n992 = global write "全局 小时数据发送次数.vi" "小时数据发送次数"(w1376) -> ()
            }
            frame True {
              n993 = global read "全局 小时数据发送次数.vi" "小时数据发送次数"() -> (w1380:i32)
              n994 = Increment(x=w1380) -> (x+1=w1379:i32)
              n995 = global write "全局 小时数据发送次数.vi" "小时数据发送次数"(w1379) -> ()
            }
          }
        }
        frame "返回执行结果" {
        }
      }
    }
    frame "提取仪器参数" {
      n996 = global read "全局1.vi" "枚举"() -> (w1384:enum16{"返回请求应答", "上传数据", "返回执行结果"})
      n997 = case shown="\"上传数据\"" w1384 {
        tunnel: ["QnRtn=1" w1394 "ExeRtn=1"] -> w1385
        tunnel: w1383 -> [_ w1392 _]
        frame "返回请求应答", Default {
          n998 = global read "全局 数据数组大小.vi" "数据数组大小"() -> (w1388:i32)
          n999 = Equal To 0?(x=w1388) -> (x = 0?=w1387:bool)
          n1000 = case shown="假" w1387 {
            frame False {
            }
            frame True {
              n1001 = global read "全局 小时数据发送次数.vi" "小时数据发送次数"() -> (w1390:i32)
              n1002 = Increment(x=w1390) -> (x+1=w1389:i32)
              n1003 = global write "全局 小时数据发送次数.vi" "小时数据发送次数"(w1389) -> ()
            }
          }
        }
        frame "上传数据" {
          n1004 = call "数据发送组合-20200825 (子VI).vi"("枚举"=T6."提取仪器参数", "插值后的数组元素"=w1392) -> ("字符串"=w1391:string)  [unwired: 9 in]
          n1005 = Empty String/Path?(string/path=w1391) -> (empty?=w1395:bool)
          n1006 = case shown="假" w1395 {
            tunnel: [w1398 ""] -> w1394
            tunnel: w1391 -> [w1398 _]
            frame False {
              n1007 = global read "全局 小时数据发送次数.vi" "小时数据发送次数"() -> (w1397:i32)
              n1008 = Increment(x=w1397) -> (x+1=w1396:i32)
              n1009 = global write "全局 小时数据发送次数.vi" "小时数据发送次数"(w1396) -> ()
            }
            frame True {
              n1010 = global read "全局 小时数据发送次数.vi" "小时数据发送次数"() -> (w1400:i32)
              n1011 = Increment(x=w1400) -> (x+1=w1399:i32)
              n1012 = global write "全局 小时数据发送次数.vi" "小时数据发送次数"(w1399) -> ()
            }
          }
        }
        frame "返回执行结果" {
        }
      }
    }
    frame "报警信息" {
      n1013 = global read "全局 小时数据发送次数.vi" "小时数据发送次数"() -> (w1405:i32)
      n1014 = Index Array(array=w1407, index (row)=w1405) -> (element=w1404:string[])  [unwired: 1 in]
      n1015 = global read "全局1.vi" "枚举"() -> (w1406:enum16{"返回请求应答", "上传数据", "返回执行结果"})
      n1016 = case shown="\"上传数据\"" w1406 {
        tunnel: ["QnRtn=1" w1420 "ExeRtn=1"] -> w1408
        tunnel: w1404 -> [_ _ _]
        tunnel: w1403 -> [_ w1415 _]
        frame "返回请求应答", Default {
          n1017 = global read "全局 数据数组大小.vi" "数据数组大小"() -> (w1411:i32)
          n1018 = Equal To 0?(x=w1411) -> (x = 0?=w1410:bool)
          n1019 = case shown="真" w1410 {
            frame False {
            }
            frame True {
              n1020 = global read "全局 小时数据发送次数.vi" "小时数据发送次数"() -> (w1413:i32)
              n1021 = Increment(x=w1413) -> (x+1=w1412:i32)
              n1022 = global write "全局 小时数据发送次数.vi" "小时数据发送次数"(w1412) -> ()
            }
          }
        }
        frame "上传数据" {
          n1023 = call "数据发送组合-20200825 (子VI).vi"("枚举"=T6."报警信息", "插值后的数组元素"=w1415) -> ("字符串"=w1414:string)  [unwired: 9 in]
          n1024 = Empty String/Path?(string/path=w1414) -> (empty?=w1421:bool)
          n1025 = String Length(string=w1414) -> (length=w1419:i32)
          n1026 = Decrement(x=w1419) -> (x-1=w1418:i32)
          n1027 = String Subset(string=w1414, length (rest)=w1418) -> (substring=w1417:string)  [unwired: 1 in]
          n1028 = case shown="假" w1421 {
            tunnel: [w1424 ""] -> w1420
            tunnel: w1417 -> [w1424 _]
            frame False {
              n1029 = global read "全局 小时数据发送次数.vi" "小时数据发送次数"() -> (w1423:i32)
              n1030 = Increment(x=w1423) -> (x+1=w1422:i32)
              n1031 = global write "全局 小时数据发送次数.vi" "小时数据发送次数"(w1422) -> ()
            }
            frame True {
              n1032 = global read "全局 小时数据发送次数.vi" "小时数据发送次数"() -> (w1426:i32)
              n1033 = Increment(x=w1426) -> (x+1=w1425:i32)
              n1034 = global write "全局 小时数据发送次数.vi" "小时数据发送次数"(w1425) -> ()
            }
          }
        }
        frame "返回执行结果" {
        }
      }
    }
    frame "系统状态" {
      # ",i12002-Info=0,i12003-Info=100,i12031-Info=0"
      # "DataTime=20100301145000;PolId=w01018,i12001-Info=1,i12003-Info=100"
      # "100  当前模式\n101  CODMn状态  （0待机，1运行）\n102  氨氮状态\n103  总磷状态\n104  总氮状态\n105  CODCr状态\n106  运行周期"
      n1035 = global read "全局 小时数据发送次数.vi" "小时数据发送次数"() -> (w1433:i32)
      n1036 = Build Array("w00000", "w01019", "w21003", "w21011", "w21001", "w01018") -> (w1436:string[])
      n1037 = global read "全局1.vi" "register values"() -> (w1434:u16[])
      n1038 = Index Array(array=w1434, index=w1433) -> (element=w1432:u16)
      n1039 = Index Array(array=w1436, index=w1433) -> (element=w1435:string)
      n1040 = case shown="1, 默认" w1433 {
        tunnel: w1435 -> [w1451 w1456]
        tunnel: w1432 -> [w1452 _]
        tunnel: [w1449 w1455] -> w1431
        frame 1, Default {
          n1041 = Number To Decimal String(number=w1452) -> (decimal integer string=w1453:string)  [unwired: 1 in]
          n1042 = Format Into String(w1453) -> (resulting string=w1450:string)  [unwired: 3 in, 1 out]
          n1043 = Format Into String(format string="PolId=%s,i12001-Info=%s,i12002-Info=0;" ("格式字符串"), w1451, w1450) -> (resulting string=w1449:string)  [unwired: 2 in, 1 out]
        }
        frame 0 {
          n1044 = Format Into String(format string="PolId=%s,i22001-Info=0,i22002-Info=1,i22003-Info=0;" ("格式字符串"), w1456) -> (resulting string=w1455:string)  [unwired: 2 in, 1 out]
        }
      }
      n1045 = Get Date/Time In Seconds() -> (seconds since 1Jan1904=w1446:timestamp)
      n1046 = Format Date/Time String(time format string (%c)="%Y%m%d%H%M%S" ("时间格式字符串(%c)"), seconds (now)=w1446) -> (date/time string=w1445:string)  [unwired: 1 in]
      n1047 = Format Into String(format string="DataTime=%s;%s" ("格式字符串"), w1445, w1431) -> (resulting string=w1442:string)  [unwired: 2 in, 1 out]
      n1048 = String Length(string=w1442) -> (length=w1444:i32)
      n1049 = Decrement(x=w1444) -> (x-1=w1443:i32)
      n1050 = String Subset(string=w1442, length (rest)=w1443) -> (substring=w1441:string)  [unwired: 1 in]
    }
    frame "运行模式" {
      # "DataTime=20100301145000;PolId=w01018,i12001-Info=1,i12003-Info=0"
      # "100  当前模式\n101  CODMn状态  （0待机，1运行）\n102  氨氮状态\n103  总磷状态\n104  总氮状态\n105  CODCr状态\n106  运行周期"
      n1051 = Get Date/Time In Seconds() -> (seconds since 1Jan1904=w1465:timestamp)
      n1052 = Format Date/Time String(time format string (%c)="%Y%m%d%H%M%S" ("时间格式字符串(%c)"), seconds (now)=w1465) -> (date/time string=w1462:string)  [unwired: 1 in]
      n1053 = global read "全局1.vi" "register values"() -> (w1467:u16[])
      n1054 = Index Array(array=w1467, index=0 ("索引")) -> (element=w1459:u16)
      n1055 = Number To Decimal String(number=w1459) -> (decimal integer string=w1461:string)  [unwired: 1 in]
      n1056 = Format Into String(format string="RunMode=%s;" ("格式字符串"), w1461) -> (resulting string=w1458:string)  [unwired: 2 in, 1 out]
      n1057 = Format Into String(format string="DataTime=%s;%s" ("格式字符串"), w1462, w1458) -> (resulting string=w1464:string)  [unwired: 2 in, 1 out]
    }
    frame "测量周期" {
      n1058 = global read "全局1.vi" "register values"() -> (w1478:u16[])
      n1059 = Index Array(array=w1478, index=6 ("索引")) -> (element=w1470:u16)
      n1060 = Get Date/Time In Seconds() -> (seconds since 1Jan1904=w1476:timestamp)
      n1061 = Format Date/Time String(time format string (%c)="%Y%m%d%H%M%S" ("时间格式字符串(%c)"), seconds (now)=w1476) -> (date/time string=w1473:string)  [unwired: 1 in]
      n1062 = Number To Decimal String(number=w1470) -> (decimal integer string=w1471:string)  [unwired: 1 in]
      n1063 = Format Into String(format string="RunInterval=%s;" ("格式字符串"), w1471) -> (resulting string=w1469:string)  [unwired: 2 in, 1 out]
      n1064 = Format Into String(format string="DataTime=%s;%s" ("格式字符串"), w1473, w1469) -> (resulting string=w1475:string)  [unwired: 2 in, 1 out]
    }
    frame "各参数测量周期" {
      # "QN=20101108135153914;ST=21;CN=2084;PW=123456;MN=A110000_0001;Flag=9;CP=&&DataTime=20100301145000;PolId=w01018,RunInterval=4;PolId=w01019,RunInterval=4;...&&"
      n1065 = global read "全局1.vi" "读取各参数测量周期的值"() -> (w1481:u16[])
      n1066 = Get Date/Time In Seconds() -> (seconds since 1Jan1904=w1484:timestamp)
      n1067 = call "2084上传各参数测量周期.vi"("读取各参数测量周期的值"=w1481) -> ("字符串"=w1480:string)  [unwired: 10 in]
      n1068 = Format Date/Time String(time format string (%c)="%Y%m%d%H%M%S" ("时间格式字符串(%c)"), seconds (now)=w1484) -> (date/time string=w1482:string)  [unwired: 1 in]
      n1069 = Format Into String(format string="DataTime=%s;%s" ("格式字符串"), w1482, w1480) -> (resulting string=w1483:string)  [unwired: 2 in, 1 out]
    }
    frame "超标留样" {
      # "DataTime=20100301145000;PolId=w01018,i12001-Info=1,i12003-Info=0"
      # "100  当前模式\n101  CODMn状态  （0待机，1运行）\n102  氨氮状态\n103  总磷状态\n104  总氮状态\n105  CODCr状态\n106  运行周期"
      n1070 = global read "全局1.vi" "register values"() -> (w1496:u16[])
      n1071 = Get Date/Time In Seconds() -> (seconds since 1Jan1904=w1494:timestamp)
      n1072 = Format Date/Time String(time format string (%c)="%Y%m%d%H%M%S" ("时间格式字符串(%c)"), seconds (now)=w1494) -> (date/time string=w1491:string)  [unwired: 1 in]
      n1073 = Index Array(array=w1496, index=7 ("索引")) -> (element=w1488:u16)
      n1074 = Number To Decimal String(number=w1488) -> (decimal integer string=w1489:string)  [unwired: 1 in]
      n1075 = Format Into String(format string="VaseNo=%s;" ("格式字符串"), w1489) -> (resulting string=w1487:string)  [unwired: 2 in, 1 out]
      n1076 = Format Into String(format string="DataTime=%s;%s" ("格式字符串"), w1491, w1487) -> (resulting string=w1493:string)  [unwired: 2 in, 1 out]
    }
    frame "3201告警信息" {
      n1077 = global read "全局 小时数据发送次数.vi" "小时数据发送次数"() -> (w1498:i32)
      n1078 = Get Date/Time In Seconds() -> (seconds since 1Jan1904=w1504:timestamp)
      n1079 = Format Date/Time String(time format string (%c)="%Y%m%d%H%M%S" ("时间格式字符串(%c)"), seconds (now)=w1504) -> (date/time string=w1502:string)  [unwired: 1 in]
      n1080 = Number To Decimal String(number=w1498) -> (decimal integer string=w1499:string)  [unwired: 1 in]
      n1081 = Format Into String(format string="SystemAlarm=%s" ("格式字符串"), w1499) -> (resulting string=w1500:string)  [unwired: 2 in, 1 out]
      n1082 = Format Into String(format string="DataTime=%s;%s" ("格式字符串"), w1502, w1500) -> (resulting string=w1503:string)  [unwired: 2 in, 1 out]
    }
  }
  n1083 = case shown="假" w24 {
    tunnel: [w1508 w1512] -> w26
    frame False {
      n1084 = global read "全局1.vi" "枚举"() -> (w1507:enum16{"返回请求应答", "上传数据", "返回执行结果"})
      n1085 = case shown="\"上传数据\"" w1507 {
        tunnel: ["91" ("CN") w1510 "91" ("CN")] -> w1508
        frame "返回请求应答", Default {
        }
        frame "上传数据" {
          n1086 = global read "全局1.vi" "系统编码ST"() -> (w1510:string)
        }
        frame "返回执行结果" {
        }
      }
    }
    frame True {
      n1087 = global read "全局 反控命令枚举.vi" "反控命令枚举"() -> (w1513:enum16{"返回请求应答", "返回执行结果"})
      n1088 = case shown="\"返回执行结果\"" w1513 {
        tunnel: ["91" "91"] -> w1512
        frame "返回请求应答", Default {
        }
        frame "返回执行结果" {
        }
      }
    }
  }
  n1089 = case shown="\"获取仪器软件版本号\"" "table输入" {
    tunnel: ["9015" ("ST") w1526 w1534 w1542 w1549 w1556 w1564 w1572 w1580 w1588 w1597 w1612 w1624 w1632 w1640 w1649 w1658 w1675 w1683 w1691 w1699 w1707 w1715 w1726 w1738 w1750 w1762 w1774 w1782 "3020" ("ST") "3042" ("ST") "3056" ("ST") "2084" ("ST") "3015" ("ST") "3201" ("ST")] -> w29
    tunnel: ["9" ("ST") "9" ("ST") "9" ("ST") "8" ("ST") "8" ("ST") "9" ("ST") "9" ("ST") "9" ("ST") "8" ("ST") "8" ("ST") "9" ("ST") "9" ("ST") "11" ("ST") "9" ("ST") "9" ("ST") w1652 "9" ("ST") "9" ("ST") "9" ("ST") "9" ("ST") "9" ("ST") "9" ("ST") "9" ("ST") "9" ("ST") "9" ("ST") "9" ("ST") "9" ("ST") "9" ("ST") "9" ("ST") "9" ("ST") "9" ("ST") "9" ("ST") "9" ("ST") "9" ("ST") "9" ("ST")] -> w28
    tunnel: w19 -> [_ w1524 w1532 w1543 w1550 w1557 w1565 w1573 w1581 w1589 w1598 w1614 w1626 w1634 w1642 w1651 w1661 w1677 w1685 w1693 w1701 w1709 w1717 w1728 w1740 w1752 w1764 w1776 w1784 w1790 w1794 w1798 w1802 w1806 w1810]
    tunnel: [_ w1524 w1532 w1543 w1550 w1557 w1565 w1573 w1581 w1589 w1598 w1614 w1626 w1634 w1642 w1651 w1661 w1677 w1685 w1693 w1701 w1709 w1717 w1728 w1740 w1752 w1764 w1776 w1784 w1790 w1794 w1798 w1802 w1806 w1810] -> w8
    tunnel: [w1516 w1523 w1531 w1539 w1547 w1554 w1562 w1570 w1578 w1586 w1594 w1611 w1623 w1631 w1639 w1648 w1660 w1673 w1681 w1689 w1697 w1705 w1713 w1721 w1733 w1745 w1757 w1769 w1781 w1789 w1793 w1797 w1801 w1805 w1809] -> w20
    tunnel: [_ _ _ _ _ _ _ _ _ _ _ _ w1621 _ _ _ _ _ _ _ _ _ _ _ _ _ _ _ _ _ _ _ _ _ _] -> w6
    tunnel: [_ _ _ _ _ _ _ _ _ _ _ _ w1619 _ _ _ _ _ _ _ _ _ _ _ _ _ _ _ _ _ _ _ _ _ _] -> w5
    frame "心跳包", Default {
      # "心跳包"
      n1090 = Get Date/Time In Seconds() -> (seconds since 1Jan1904=w1519:timestamp)
      n1091 = Format Date/Time String(time format string (%c)="%Y%m%d%H%M%S%3u" ("时间格式字符串(%c)"), seconds (now)=w1519) -> (date/time string=w1518:string)  [unwired: 1 in]
      n1092 = Search and Replace String(input string=w1518, search string="." ("搜索字符串")) -> (result string=w1516:string)  [unwired: 6 in, 3 out]
    }
    frame "提取数采仪时间" {
      n1093 = global read "全局1.vi" "枚举"() -> (w1527:enum16{"返回请求应答", "上传数据", "返回执行结果"})
      n1094 = case shown="\"返回执行结果\"" w1527 {
        tunnel: ["9011" ("CN") "1014" ("CN") "9012" ("CN")] -> w1526
        frame "返回请求应答", Default {
        }
        frame "上传数据" {
        }
        frame "返回执行结果" {
        }
      }
      n1095 = local read "QN"() -> (w1523:string)
    }
    frame "提取实时数据间隔" {
      n1096 = global read "全局1.vi" "枚举"() -> (w1535:enum16{"返回请求应答", "上传数据", "返回执行结果"})
      n1097 = case shown="\"上传数据\"" w1535 {
        tunnel: ["9011" ("CN") "1061" ("CN") "9012" ("CN")] -> w1534
        frame "返回请求应答", Default {
        }
        frame "上传数据" {
        }
        frame "返回执行结果" {
        }
      }
      n1098 = local read "QN"() -> (w1531:string)
    }
    frame "反控命令" {
      n1099 = global read "全局 反控命令枚举.vi" "反控命令枚举"() -> (w1540:enum16{"返回请求应答", "返回执行结果"})
      n1100 = case shown="\"返回请求应答\", 默认" w1540 {
        tunnel: ["9011" ("CN") "9012" ("CN")] -> w1542
        frame "返回请求应答", Default {
        }
        frame "返回执行结果" {
        }
      }
      n1101 = local read "QN"() -> (w1539:string)
    }
    frame "超标留样返回" {
      n1102 = global read "全局1.vi" "枚举"() -> (w1546:enum16{"返回请求应答", "上传数据", "返回执行结果"})
      n1103 = case shown="\"上传数据\"" w1546 {
        tunnel: ["9011" ("CN") "3015" ("CN") "9012" ("CN")] -> w1549
        frame "返回请求应答", Default {
        }
        frame "上传数据" {
        }
        frame "返回执行结果" {
        }
      }
      n1104 = local read "QN"() -> (w1547:string)
    }
    frame "提取经纬度环境信息" {
      n1105 = global read "全局1.vi" "枚举"() -> (w1558:enum16{"返回请求应答", "上传数据", "返回执行结果"})
      n1106 = case shown="\"上传数据\"" w1558 {
        tunnel: ["9011" ("CN") "3041" ("CN") "9012" ("CN")] -> w1556
        frame "返回请求应答", Default {
        }
        frame "上传数据" {
        }
        frame "返回执行结果" {
        }
      }
      n1107 = local read "QN"() -> (w1554:string)
    }
    frame "提取现场系统信息" {
      n1108 = global read "全局1.vi" "枚举"() -> (w1566:enum16{"返回请求应答", "上传数据", "返回执行结果"})
      n1109 = case shown="\"上传数据\"" w1566 {
        tunnel: ["9011" ("CN") "3040" ("CN") "9012" ("CN")] -> w1564
        frame "返回请求应答", Default {
        }
        frame "上传数据" {
        }
        frame "返回执行结果" {
        }
      }
      n1110 = local read "QN"() -> (w1562:string)
    }
    frame "提取监测仪表时间" {
      n1111 = global read "全局1.vi" "枚举"() -> (w1574:enum16{"返回请求应答", "上传数据", "返回执行结果"})
      n1112 = case shown="\"上传数据\"" w1574 {
        tunnel: ["9011" ("CN") "1011" ("CN") "9012" ("CN")] -> w1572
        frame "返回请求应答", Default {
        }
        frame "上传数据" {
        }
        frame "返回执行结果" {
        }
      }
      n1113 = local read "QN"() -> (w1570:string)
    }
    frame "获取软件版本号" {
      n1114 = global read "全局1.vi" "枚举"() -> (w1582:enum16{"返回请求应答", "上传数据", "返回执行结果"})
      n1115 = case shown="\"返回执行结果\"" w1582 {
        tunnel: ["9011" ("CN") "3100" ("CN") "9012" ("CN")] -> w1580
        frame "返回请求应答", Default {
        }
        frame "上传数据" {
        }
        frame "返回执行结果" {
        }
      }
      n1116 = local read "QN"() -> (w1578:string)
    }
    frame "获取仪器软件版本号" {
      n1117 = global read "全局1.vi" "枚举"() -> (w1590:enum16{"返回请求应答", "上传数据", "返回执行结果"})
      n1118 = case shown="\"上传数据\"" w1590 {
        tunnel: ["9011" ("CN") "3102" ("CN") "9012" ("CN")] -> w1588
        frame "返回请求应答", Default {
        }
        frame "上传数据" {
        }
        frame "返回执行结果" {
        }
      }
      n1119 = local read "QN"() -> (w1586:string)
    }
    frame "实时数据" {
      n1120 = global read "全局1.vi" "枚举"() -> (w1596:enum16{"返回请求应答", "上传数据", "返回执行结果"})
      n1121 = case shown="\"上传数据\"" w1596 {
        tunnel: ["9011" ("CN") w1601 "9012" ("CN")] -> w1597
        frame "返回请求应答", Default {
        }
        frame "上传数据" {
          n1122 = global read "全局 实时数据参数.vi" "实时数据参数"() -> (w1600:string)
          n1123 = case shown="\"平行样测试\"" w1600 {
            tunnel: ["2011" ("CN") "2064" ("CN") "2082" ("CN") "2063" ("CN") "2062" ("CN") "2065" ("CN") "2066" ("CN") "fff" ("CN")] -> w1601
            frame "水样测试", Default {
            }
            frame "平行样测试" {
            }
            frame "集成干预测试" {
            }
            frame "加标回收测试" {
            }
            frame "核查数据" {
            }
            frame "空白测试" {
            }
            frame "跨度核查" {
            }
            frame "" {
            }
          }
        }
        frame "返回执行结果" {
        }
      }
      n1124 = local read "QN"() -> (w1594:string)
    }
    frame "小时数据" {
      # "监测小时数据"
      n1125 = global read "全局1.vi" "枚举"() -> (w1613:enum16{"返回请求应答", "上传数据", "返回执行结果"})
      n1126 = case shown="\"上传数据\"" w1613 {
        tunnel: ["9011" ("CN") "2061" ("CN") "9012" ("CN")] -> w1612
        frame "返回请求应答", Default {
        }
        frame "上传数据" {
        }
        frame "返回执行结果" {
        }
      }
      n1127 = local read "QN"() -> (w1611:string)
    }
    frame "剖面数据" {
      n1128 = global read "全局1.vi" "枚举"() -> (w1625:enum16{"返回请求应答", "上传数据", "返回执行结果"})
      n1129 = case shown="\"上传数据\"" w1625 {
        tunnel: ["9011" ("CN") "2083" ("CN") "9012" ("CN")] -> w1624
        frame "返回请求应答", Default {
        }
        frame "上传数据" {
        }
        frame "返回执行结果" {
        }
      }
      n1130 = global read "全局 数据数组大小.vi" "当前包号"() -> (w1620:i32)
      n1131 = global read "全局 数据数组大小.vi" "总包数"() -> (w1622:i32)
      n1132 = Number To Decimal String(number=w1622) -> (decimal integer string=w1621:string)  [unwired: 1 in]
      n1133 = Number To Decimal String(number=w1620) -> (decimal integer string=w1619:string)  [unwired: 1 in]
      n1134 = local read "QN"() -> (w1623:string)
    }
    frame "剖面多参数H" {
      # "监测小时数据"
      n1135 = global read "全局1.vi" "枚举"() -> (w1633:enum16{"返回请求应答", "上传数据", "返回执行结果"})
      n1136 = case shown="\"上传数据\"" w1633 {
        tunnel: ["9011" ("CN") "2061" ("CN") "9012" ("CN")] -> w1632
        frame "返回请求应答", Default {
        }
        frame "上传数据" {
        }
        frame "返回执行结果" {
        }
      }
      n1137 = local read "QN"() -> (w1631:string)
    }
    frame "剖面多参数S" {
      # "监测小时数据"
      n1138 = global read "全局1.vi" "枚举"() -> (w1641:enum16{"返回请求应答", "上传数据", "返回执行结果"})
      n1139 = case shown="\"上传数据\"" w1641 {
        tunnel: ["9011" ("CN") "2011" ("CN") "9012" ("CN")] -> w1640
        frame "返回请求应答", Default {
        }
        frame "上传数据" {
        }
        frame "返回执行结果" {
        }
      }
      n1140 = local read "QN"() -> (w1639:string)
    }
    frame "提取小时数据" {
      # "监测小时数据"
      n1141 = global read "全局1.vi" "枚举"() -> (w1650:enum16{"返回请求应答", "上传数据", "返回执行结果"})
      n1142 = global read "断电保存全局.vi" "数据组合发送"() -> (w1647:bool)
      n1143 = case shown="\"上传数据\"" w1650 {
        tunnel: ["9011" ("CN") "2061" ("CN") "9012" ("CN")] -> w1649
        frame "返回请求应答", Default {
        }
        frame "上传数据" {
        }
        frame "返回执行结果" {
        }
      }
      n1144 = case shown="假" w1647 {
        tunnel: ["9" ("ST") "9" ("ST")] -> w1652
        frame False {
        }
        frame True {
        }
      }
      n1145 = local read "QN"() -> (w1648:string)
    }
    frame "提取实时数据" {
      # "提取实时数据"
      n1146 = global read "全局1.vi" "枚举"() -> (w1659:enum16{"返回请求应答", "上传数据", "返回执行结果"})
      n1147 = case shown="\"上传数据\"" w1659 {
        tunnel: ["9011" ("CN") w1665 "9012" ("CN")] -> w1658
        frame "返回请求应答", Default {
        }
        frame "上传数据" {
          n1148 = global read "全局 实时数据参数.vi" "实时数据参数"() -> (w1664:string)
          n1149 = case shown="\"平行样测试\"" w1664 {
            tunnel: ["2011" ("CN") "2064" ("CN") "2063" ("CN") "2065" ("CN") "2066" ("CN") "fff" ("CN")] -> w1665
            frame "水样测试", Default {
            }
            frame "平行样测试" {
            }
            frame "加标回收测试" {
            }
            frame "空白测试" {
            }
            frame "跨度核查" {
            }
            frame "" {
            }
          }
        }
        frame "返回执行结果" {
        }
      }
      n1150 = local read "QN"() -> (w1660:string)
    }
    frame "跨度核查" {
      # "跨度核查"
      n1151 = global read "全局1.vi" "枚举"() -> (w1676:enum16{"返回请求应答", "上传数据", "返回执行结果"})
      n1152 = case shown="\"上传数据\"" w1676 {
        tunnel: ["9011" ("CN") "2066" ("ST") "9012" ("CN")] -> w1675
        frame "返回请求应答", Default {
        }
        frame "上传数据" {
        }
        frame "返回执行结果" {
        }
      }
      n1153 = local read "QN"() -> (w1673:string)
    }
    frame "提取加标回收" {
      # "提取加标回收"
      n1154 = global read "全局1.vi" "枚举"() -> (w1684:enum16{"返回请求应答", "上传数据", "返回执行结果"})
      n1155 = case shown="\"上传数据\"" w1684 {
        tunnel: ["9011" ("CN") "2063" ("ST") "9012" ("CN")] -> w1683
        frame "返回请求应答", Default {
        }
        frame "上传数据" {
        }
        frame "返回执行结果" {
        }
      }
      n1156 = local read "QN"() -> (w1681:string)
    }
    frame "提取平行样" {
      # "提取平行样"
      n1157 = global read "全局1.vi" "枚举"() -> (w1692:enum16{"返回请求应答", "上传数据", "返回执行结果"})
      n1158 = case shown="\"上传数据\"" w1692 {
        tunnel: ["9011" ("CN") "2064" ("ST") "9012" ("CN")] -> w1691
        frame "返回请求应答", Default {
        }
        frame "上传数据" {
        }
        frame "返回执行结果" {
        }
      }
      n1159 = local read "QN"() -> (w1689:string)
    }
    frame "空白测试", "零点核查" {
      # "零点核查"
      n1160 = global read "全局1.vi" "枚举"() -> (w1700:enum16{"返回请求应答", "上传数据", "返回执行结果"})
      n1161 = case shown="\"上传数据\"" w1700 {
        tunnel: ["9011" ("CN") "2065" ("ST") "9012" ("CN")] -> w1699
        frame "返回请求应答", Default {
        }
        frame "上传数据" {
        }
        frame "返回执行结果" {
        }
      }
      n1162 = local read "QN"() -> (w1697:string)
    }
    frame "核查数据" {
      # "核查数据"
      n1163 = global read "全局1.vi" "枚举"() -> (w1708:enum16{"返回请求应答", "上传数据", "返回执行结果"})
      n1164 = case shown="\"上传数据\"" w1708 {
        tunnel: ["9011" ("CN") "2062" ("ST") "9012" ("CN")] -> w1707
        frame "返回请求应答", Default {
        }
        frame "上传数据" {
        }
        frame "返回执行结果" {
        }
      }
      n1165 = local read "QN"() -> (w1705:string)
    }
    frame "提取集成干预" {
      # "核查数据"
      n1166 = global read "全局1.vi" "枚举"() -> (w1716:enum16{"返回请求应答", "上传数据", "返回执行结果"})
      n1167 = case shown="\"上传数据\"" w1716 {
        tunnel: ["9011" ("CN") "2082" ("ST") "9012" ("CN")] -> w1715
        frame "返回请求应答", Default {
        }
        frame "上传数据" {
        }
        frame "返回执行结果" {
        }
      }
      n1168 = local read "QN"() -> (w1713:string)
    }
    frame "报警信息", "采配水仪器参数", "操作日志", "仪器参数" {
      n1169 = global read "全局1.vi" "枚举"() -> (w1727:enum16{"返回请求应答", "上传数据", "返回执行结果"})
      n1170 = case shown="\"上传数据\"" w1727 {
        tunnel: ["9011" ("CN") "3020" ("CN") "9012" ("CN")] -> w1726
        frame "返回请求应答", Default {
        }
        frame "上传数据" {
        }
        frame "返回执行结果" {
        }
      }
      n1171 = Get Date/Time In Seconds() -> (seconds since 1Jan1904=w1724:timestamp)
      n1172 = Format Date/Time String(time format string (%c)="%Y%m%d%H%M%S%3u" ("时间格式字符串(%c)"), seconds (now)=w1724) -> (date/time string=w1723:string)  [unwired: 1 in]
      n1173 = Search and Replace String(input string=w1723, search string="." ("搜索字符串")) -> (result string=w1721:string)  [unwired: 6 in, 3 out]
    }
    frame "3092日志信息" {
      n1174 = global read "全局1.vi" "枚举"() -> (w1739:enum16{"返回请求应答", "上传数据", "返回执行结果"})
      n1175 = case shown="\"上传数据\"" w1739 {
        tunnel: ["9011" ("CN") "3092" ("CN") "9012" ("CN")] -> w1738
        frame "返回请求应答", Default {
        }
        frame "上传数据" {
        }
        frame "返回执行结果" {
        }
      }
      n1176 = Get Date/Time In Seconds() -> (seconds since 1Jan1904=w1736:timestamp)
      n1177 = Format Date/Time String(time format string (%c)="%Y%m%d%H%M%S%3u" ("时间格式字符串(%c)"), seconds (now)=w1736) -> (date/time string=w1735:string)  [unwired: 1 in]
      n1178 = Search and Replace String(input string=w1735, search string="." ("搜索字符串")) -> (result string=w1733:string)  [unwired: 6 in, 3 out]
    }
    frame "3093报警信息" {
      n1179 = global read "全局1.vi" "枚举"() -> (w1751:enum16{"返回请求应答", "上传数据", "返回执行结果"})
      n1180 = case shown="\"上传数据\"" w1751 {
        tunnel: ["9011" ("CN") "3093" ("CN") "9012" ("CN")] -> w1750
        frame "返回请求应答", Default {
        }
        frame "上传数据" {
        }
        frame "返回执行结果" {
        }
      }
      n1181 = Get Date/Time In Seconds() -> (seconds since 1Jan1904=w1748:timestamp)
      n1182 = Format Date/Time String(time format string (%c)="%Y%m%d%H%M%S%3u" ("时间格式字符串(%c)"), seconds (now)=w1748) -> (date/time string=w1747:string)  [unwired: 1 in]
      n1183 = Search and Replace String(input string=w1747, search string="." ("搜索字符串")) -> (result string=w1745:string)  [unwired: 6 in, 3 out]
    }
    frame "3090仪器参数" {
      n1184 = global read "全局1.vi" "枚举"() -> (w1763:enum16{"返回请求应答", "上传数据", "返回执行结果"})
      n1185 = case shown="\"上传数据\"" w1763 {
        tunnel: ["9011" ("CN") "3090" ("CN") "9012" ("CN")] -> w1762
        frame "返回请求应答", Default {
        }
        frame "上传数据" {
        }
        frame "返回执行结果" {
        }
      }
      n1186 = Get Date/Time In Seconds() -> (seconds since 1Jan1904=w1760:timestamp)
      n1187 = Format Date/Time String(time format string (%c)="%Y%m%d%H%M%S%3u" ("时间格式字符串(%c)"), seconds (now)=w1760) -> (date/time string=w1759:string)  [unwired: 1 in]
      n1188 = Search and Replace String(input string=w1759, search string="." ("搜索字符串")) -> (result string=w1757:string)  [unwired: 6 in, 3 out]
    }
    frame "3091校准信息" {
      n1189 = global read "全局1.vi" "枚举"() -> (w1775:enum16{"返回请求应答", "上传数据", "返回执行结果"})
      n1190 = case shown="\"上传数据\"" w1775 {
        tunnel: ["9011" ("CN") "3091" ("CN") "9012" ("CN")] -> w1774
        frame "返回请求应答", Default {
        }
        frame "上传数据" {
        }
        frame "返回执行结果" {
        }
      }
      n1191 = Get Date/Time In Seconds() -> (seconds since 1Jan1904=w1772:timestamp)
      n1192 = Format Date/Time String(time format string (%c)="%Y%m%d%H%M%S%3u" ("时间格式字符串(%c)"), seconds (now)=w1772) -> (date/time string=w1771:string)  [unwired: 1 in]
      n1193 = Search and Replace String(input string=w1771, search string="." ("搜索字符串")) -> (result string=w1769:string)  [unwired: 6 in, 3 out]
    }
    frame "提取仪器参数" {
      n1194 = global read "全局1.vi" "枚举"() -> (w1783:enum16{"返回请求应答", "上传数据", "返回执行结果"})
      n1195 = case shown="\"上传数据\"" w1783 {
        tunnel: ["9011" ("CN") "3020" ("CN") "9012" ("CN")] -> w1782
        frame "返回请求应答", Default {
        }
        frame "上传数据" {
        }
        frame "返回执行结果" {
        }
      }
      n1196 = local read "QN"() -> (w1781:string)
    }
    frame "系统状态" {
      n1197 = local read "QN"() -> (w1789:string)
    }
    frame "运行模式" {
      n1198 = local read "QN"() -> (w1793:string)
    }
    frame "测量周期" {
      n1199 = local read "QN"() -> (w1797:string)
    }
    frame "各参数测量周期" {
      n1200 = local read "QN"() -> (w1801:string)
    }
    frame "超标留样" {
      n1201 = local read "QN"() -> (w1805:string)
    }
    frame "3201告警信息" {
      n1202 = local read "QN"() -> (w1809:string)
    }
  }
  n1203 = Bundle By Name(cluster="数据块", "ST"=w26, "CN"=w29, "FLAG"=w28, "CP"=w8, "QN"=w20, "MN"="MN", "PW"="PW", "PNUM"=w6, "PNO"=w5) -> (w27:T1)
  n1204 = call "HJ212-2017.vi"("PWD？"=FALSE, "数据段"=w27) -> ("通讯包字符串"=w1:string, "通讯包"=→"通讯包":T2)  [unwired: 7 in, 1 out]
  "通讯包字符串" <- w1
  n1205 = String Length(string=w1) -> (length=→"长度":i32)
  "错误常量" <- "错误常量 2"
  "小时数据发送次数" <- 0 ("小时数据发送次数")
  "核查数据发送次数" <- 0 ("核查数据发送次数")
